vi "FL24 Dryer Tool Main.vi"() -> ()   [LabVIEW 2016]
uses:
  Common/LabVIEW GEA2 Toolkit/LabVIEW_GEA2_Toolkit.lvlibp/type defs/Data In.ctl
  Common/LabVIEW GEA2 Toolkit/LabVIEW_GEA2_Toolkit.lvlibp/type defs/Source_Destination.ctl
  Common/LabVIEW GEA2 Toolkit/LabVIEW_GEA2_Toolkit.lvlibp/type defs/Data Type.ctl
  Common/LabVIEW GEA2 Toolkit/LabVIEW_GEA2_Toolkit.lvlibp/type defs/ERD Read Data In.ctl
  Laundry Tool 2.0 Support/type defs2/Select _Graph_Brass.ctl
  Laundry Tool 1.0 Support/type defs/ERD_Graph_All.ctl
  Laundry Tool 1.0 Support/type defs/ERD_Graph.ctl
  Laundry Tool 1.0 Support/type defs/Version.ctl
  Laundry Tool 2.0 Support/type defs2/ERD_Always_Show_Brass.ctl
  Laundry Tool 1.0 Support/type defs/Fault_Buffer_Status.ctl
  Laundry Tool 2.0 Support/type defs2/Diagnostics_Table.ctl
  Laundry Tool 1.0 Support/type defs/Cycle_Diag_Buffer_Status.ctl
  Laundry Tool 2.0 Support/type defs2/ERD_Data_Loop_Control_Brass.ctl
  Laundry Tool 2.0 Support/type defs2/ERD_Loop_States_Brass.ctl
  Laundry Tool 2.0 Support/type defs2/Error_Command_Brass.ctl
  Laundry Tool 2.0 Support/type defs2/DAQ_States_Brass.ctl
  Common/GExplorer Support/typedefs/GExplorer_Data_Cluster.ctl
  Laundry Tool 1.0 Support/type defs/Cont_Send_States.ctl
  Laundry Tool 2.0 Support/type defs2/Cont_Send_States_Brass.ctl
  Common/LabVIEW GEA2 Toolkit/LabVIEW_GEA2_Toolkit.lvlibp/type defs/Data Out.ctl
  Common/LabVIEW GEA2 Toolkit/LabVIEW_GEA2_Toolkit.lvlibp/type defs/ERD Write Data In.ctl
  Laundry Tool 2.0 Support/type defs2/DAQ_Control_Command_Brass.ctl
  Laundry Tool 2.0 Support/type defs2/ERD_Loop_Control_Command_Brass.ctl
  Laundry Tool 2.0 Support/type defs2/GEA2_Control_Command_Brass.ctl
  <vilib>/DAQmx/read.llb/DAQmx Read (Digital 1D Bool NChan 1Samp 1Line).vi
  <vilib>/DAQmx/read.llb/DAQmx Read (Digital 1D U8 1Chan NSamp).vi
  <vilib>/DAQmx/write.llb/DAQmx Write (Digital Bool 1Line 1Point).vi
  <vilib>/DAQmx/read.llb/DAQmx Read (Counter U32 1Chan 1Samp).vi
  <vilib>/DAQmx/write.llb/DAQmx Write (Analog 1D DBL NChan 1Samp).vi
  <vilib>/DAQmx/write.llb/DAQmx Write (Digital 1D Bool NChan 1Samp 1Line).vi
  Common/LabVIEW GEA2 Toolkit/LabVIEW_GEA2_Toolkit.lvlibp/advanced/GEA2 Message Received Event Handler.vi
  <vilib>/DAQmx/create/channels.llb/DAQmx Create Channel (DO-Digital Output).vi
  <vilib>/DAQmx/create/channels.llb/DAQmx Create Channel (DI-Digital Input).vi
  <vilib>/DAQmx/configure/timing.llb/DAQmx Timing (Sample Clock).vi
  <vilib>/DAQmx/create/channels.llb/DAQmx Create Channel (CO-Pulse Generation-Frequency).vi
  <vilib>/DAQmx/configure/timing.llb/DAQmx Timing (Implicit).vi
  <vilib>/DAQmx/create/channels.llb/DAQmx Create Channel (CI-Count Edges).vi
  <vilib>/DAQmx/create/channels.llb/DAQmx Create Channel (AO-Voltage-Basic).vi
  <vilib>/DAQmx/miscellaneous.llb/DAQmx Fill In Error Info.vi
  C:/Automation/DLLs/PC Dot Net/GeaCommunication.dll
  Common/LabVIEW GEA2 Toolkit/LabVIEW_GEA2_Toolkit.lvlibp
  Automation/Product Specific/Clothes Care/2015 VA Washer/Projects/2015 VA Washer.lvlib
  <resource>/objmgr/daqmx.rc
panel:
  in  "Data ON":bool=TRUE
  out "ERD_Always Show":T1
  in  "Stop":bool
  out "Fault Status":bool
  out "Log Rate (ms)":u32
  in  "Tab Control":T2(tab)
  in  "Filter Data":bool=TRUE
  in  "Start Send":bool
  in  "Cmd":string
  in  "Filter Log":bool
  in  "Msg Rate (ms)":u32=1000 min=50 step=50
  out "CSV File Log Path":path=path "C:/Users/502129737/Desktop/1"
  in  "Clear":bool
  out "GEA2 Log":string
  in  "Board Index":u8 max=0 step=1
  out "Board ID":string="0"
  in  "GEA2 Send":T3={"Source"=228, "Destination"=53, "Command"=0, "Message"=""} {"Command" format="%02x"; "Destination" format="%02x"; "Source" format="%02x"}
  in  "Send Button":bool
  in  "GEA2 Log Length":i32=100000
  in  "Save Log":bool
  out "Version":T4
  in  "GEA Inputs":T5={"Source"=228, "Destination"=53} {"Destination" format="%.0x"; "Source" format="%.0x"}
  in  "Read ERD List":T6[](array[typedef])=[{"ERD Number"=0, "Data Type"=enum."string"}] {"ERD Number" format="%.0x"}
  out "Read ERD Data Out":cluster{"ERD Number":u16, "Data":string}[](array[cluster]) {"ERD Number" format="%.0x"}
  in  "Read ERD":bool
  in  "Write ERD":bool
  in  "Write ERD List":T8(array[cluster])=[{"ERD Number"=0, "Data Type"=enum."string", "Data"=""}] {"ERD Number" format="%.0x"}
  in  "Graphing ON":bool=TRUE
  in  "Select Graph":T9
  out "ERD 3":dbl(graph)
  out "ERD 2":dbl(graph)
  out "ERD 1":dbl(graph)
  out "All Loads":u16[][](graph)
  in  "ERD Graphing ON":bool
  out "ERD Graph  Ind":T10
  in  "ERD Graph Cntrl":T11={"ERD 3"={"ERD #"=142, "Data Type"=enum."uint32_t", "Scaler"=32}, "ERD 2"={"ERD #"=142, "Data Type"=enum."uint32_t", "Scaler"=32}, "ERD 1"={"ERD #"=142, "Data Type"=enum."int32_t", "Scaler"=32}} {"ERD 1"."Scaler" min=1; "ERD 1"."ERD #" format="%.0x"; "ERD 2"."Scaler" min=1; "ERD 2"."ERD #" format="%.0x"; "ERD 3"."Scaler" min=1; "ERD 3"."ERD #" format="%.0x"}
  in  "Save Fault Log":bool
  in  "Clear Fault Table Buffer":bool
  in  "Clear Fault Seq Buffer":bool
  in  "Fault ON":bool
  out "Fault Table Buffer":string[][](table)
  out "Fault Sequence Buffer":string
  out "Seq Buffer Status":T13
  out "Table Buffer Status":T13
  in  "Save Cycle History Log":bool
  in  "Clear Cycle Buffer":bool
  out "Cycle Buffer Status":T14
  in  "Get Cycle History":bool
  out "Diagnostics Table":T15
  in  "Test Mode":cluster{"Exit":bool, "Enter":bool}
  in  "Drum Light":cluster{"ON":bool, "OFF":bool}
  in  "Motor":cluster{"CW":bool, "OFF":bool, "CCW":bool}
  in  "Heaters":T16
  in  "Pump":cluster{"ON":bool, "OFF":bool}
  in  "Main Relay":cluster{"ON":bool, "OFF":bool}
  in  "Buzzer":cluster{"ON":bool, "OFF":bool}
  in  "LEDs":cluster{"ON":bool, "OFF":bool}
  in  "HE/LE ?":enum16{"HE", "LE"}(ring)
  in  "LL (M - A)":bool=TRUE
  in  "Lid Lock Feedback":bool
  in  "MS (M - A)":bool=TRUE
  out "DAQ Status":string
  out "Drain Pump":bool
  out "Mode Shift":bool
  out "Recirc Pump":bool
  out "Cold Valve":bool
  out "Hot Valve":bool
  out "Spray/Rinse Valve":bool
  out "Fabric SoftValve":bool
  in  "AC Power":bool=TRUE
  in  "Mode Shift FB":bool
  in  "Lid Status":bool=TRUE
  in  "Pressure":dbl(slide) min=0.0 max=5.0 step=0.5 scale=0.0..5.0 scale format="%#_3g"
  in  "Motor Current":dbl(slide)=2.5 min=0.0 max=5.0 step=0.5 scale=0.0..5.0 scale format="%#_3g"
  in  "Turn On DAQ":bool
  out "DAQ On?":bool
  in  "Basket RPM":dbl=1.0 min=1.0 max=800.0 step=5.0
  in  "Temperature":dbl(slide)=2.5 min=0.0 max=5.0 step=0.5 scale=0.0..5.0 scale format="%#_3g"
  out "Triac CW":bool
  out "Traic CCW":bool
  out "CCW":u32
  out "CW":u32
  in  "ERD Read List":T17(array[cluster])=[{"Boolean"=TRUE, "ERD Number"=1, "ERD Name"="Model Number", "Data Type"=enum."string"}, {"Boolean"=TRUE, "ERD Number"=2, "ERD Name"="Serial Number", "Data Type"=enum."string"}, {"Boolean"=TRUE, "ERD Number"=8192, "ERD Name"="Machine Status", "Data Type"=enum."uint8_t"}, {"Boolean"=TRUE, "ERD Number"=8202, "ERD Name"="Cycle Name", "Data Type"=enum."string"}, {"Boolean"=TRUE, "ERD Number"=142, "ERD Name"="Cycle Count", "Data Type"=enum."uint32_t"}, {"Boolean"=TRUE, "ERD Number"=8193, "ERD Name"="Sub-Cycle", "Data Type"=enum."string"}, {"Boolean"=TRUE, "ERD Number"=141, "ERD Name"="System Runtime", "Data Type"=enum."uint32_t"}, {"Boolean"=TRUE, "ERD Number"=8208, "ERD Name"="Delay Time", "Data Type"=enum."uint16_t"}, {"Boolean"=FALSE, "ERD Number"=256, "ERD Name"="Version", "Data Type"=enum."string"}, {"Boolean"=TRUE, "ERD Number"=70, "ERD Name"="Cycle Time", "Data Type"=enum."uint16_t"}, {"Boolean"=TRUE, "ERD Number"=8206, "ERD Name"="Operating Mode", "Data Type"=enum."string"}, {"Boolean"=TRUE, "ERD Number"=8217, "ERD Name"="Temp Level", "Data Type"=enum."string"}, {"Boolean"=TRUE, "ERD Number"=8218, "ERD Name"="Dryness Level", "Data Type"=enum."string"}, {"Boolean"=TRUE, "ERD Number"=8219, "ERD Name"="Extended Tumble", "Data Type"=enum."string"}, {"Boolean"=TRUE, "ERD Number"=61447, "ERD Name"="Input Status", "Data Type"=enum."string"}, {"Boolean"=TRUE, "ERD Number"=61448, "ERD Name"="Dryer Type", "Data Type"=enum."string"}, {"Boolean"=TRUE, "ERD Number"=8220, "ERD Name"="Cycle Type", "Data Type"=enum."string"}, {"Boolean"=TRUE, "ERD Number"=61449, "ERD Name"="Software Version", "Data Type"=enum."string"}] {"ERD Number" format="%.0x"}
  out "Error Out":errorcluster
  in  "Error In":errorcluster
  # "UI: 0x35\nMC: 0x2C"
  # "Software Version"
  # "UI - Critical Version"
  # "UI - Non-Critical"
  # "MC -  Version"
  # "Diagnostic Data Version"
  # "Model Setting"
  # "Heater Type"
  # "Must input a valid ERD# and Data Type\nDO NOT Leave Blank \nIf no scaler use value of 01"
  # "Contact:\n\nDerek Hibdon\nderek.hibdon@ge.com"
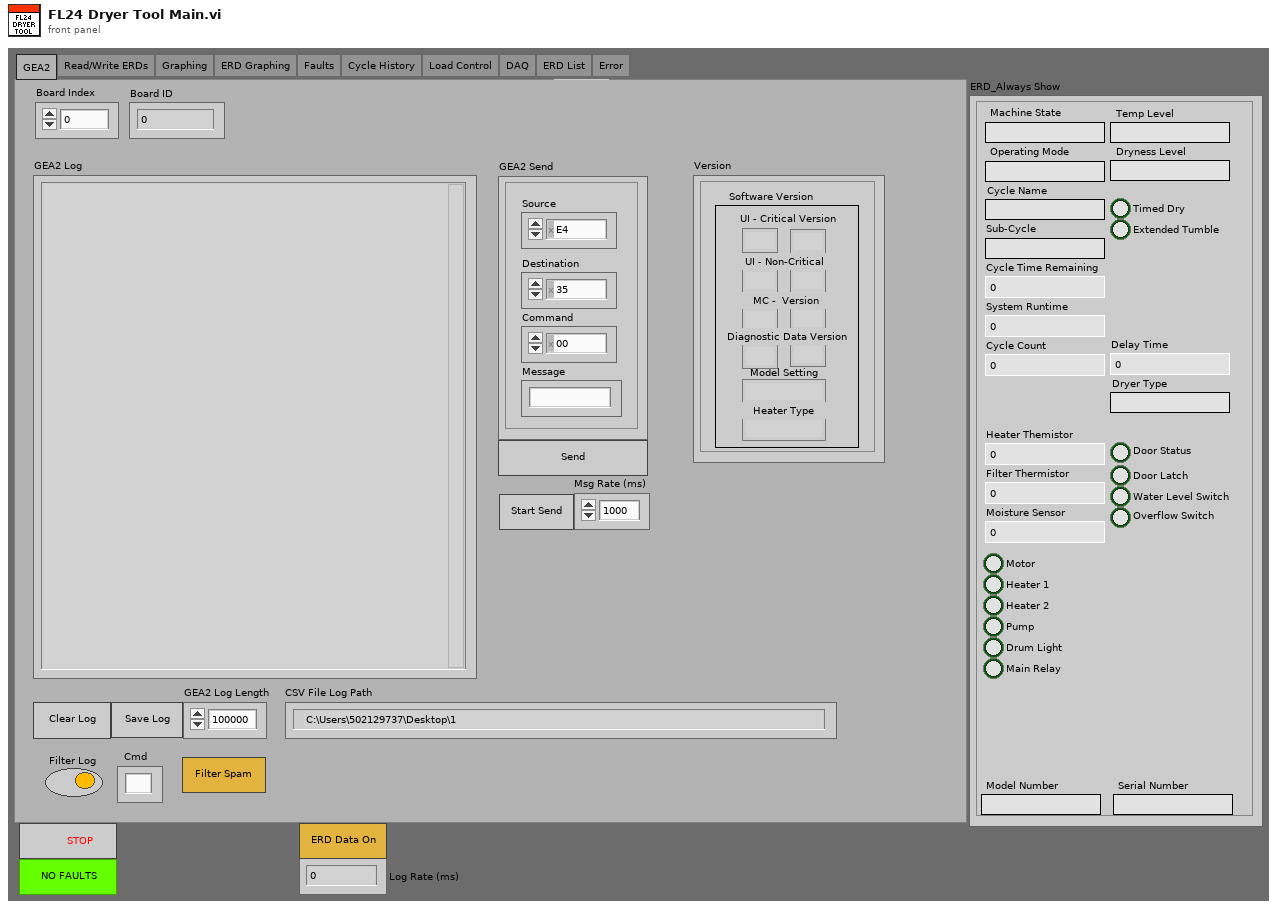
[diagram p1: front panel]
types:
  T1 = typedef "ERD_Always_Show_Brass.ctl" = cluster{"Machine State":string, "Cycle Count":u32, "Dryness Level":string, "Temp Level":string, "Delay Time":u16, "Sub-Cycle":string, "Cycle Name":string, "Model Number":string, "Serial Number":string, "System Runtime":u32, "Cycle Time Remaining":u16, "Operating Mode":string, "Heater Themistor":u16, "Water Level Switch":bool, "Overflow Switch":bool, "Door Status":bool, "Door Latch":bool, "Heater 1":bool, "Filter Thermistor":u16, "Moisture Sensor":u16, "Dryer Type":string, "Timed Dry":bool, "Extended Tumble":bool, "Heater 2":bool, "Pump":bool, "Drum Light":bool, "Main Relay":bool, "Motor":bool}
  T2 = enum32{"GEA2", "Read/Write ERDs", "Graphing", "ERD Graphing", "Faults", "Cycle History", "Load Control", "DAQ", "ERD List", "Error"}
  T3 = typedef "LabVIEW_GEA2_Toolkit.lvlibp/Data In.ctl" = cluster{"Source":u8, "Destination":u8, "Command":u8, "Message":string}
  T4 = typedef "Version.ctl" = cluster{"UI - Critical Major":string, "UI - Critical Minor":string, "UI - Non-Critical Minor":string, "UI - Non-Critical Major":string, "MC Minor":string, "MC Major":string, "Model Setting":string, "Diagnostic Data Minor":string, "Diagnostic Data Major":string, "Heater Type":string}
  T5 = typedef "LabVIEW_GEA2_Toolkit.lvlibp/Source_Destination.ctl" = cluster{"Source":u8, "Destination":u8}
  T6 = typedef "LabVIEW_GEA2_Toolkit.lvlibp/ERD Read Data In.ctl" = cluster{"ERD Number":u16, "Data Type":T7}
  T7 = typedef "LabVIEW_GEA2_Toolkit.lvlibp/Data Type.ctl" = enum16{"string", "boolean", "uint8_t", "uint16_t", "uint32_t", "uint64_t", "int8_t", "int16_t", "int32_t", "int64_t"}
  T8 = cluster{"ERD Number":u16, "Data Type":T7, "Data":string}[]
  T9 = typedef "Select _Graph_Brass.ctl" = enum16{"All Loads", "ERD 1", "ERD 2", "ERD 3", "Temperature (F)", "Basket Speed (RPM)", "Tub Volume (Gal)", "Pressure (in H2O)", "Current RMS (Amps)"}
  T10 = cluster{"ERD Value 1":dbl, "ERD Value 2":dbl, "ERD Value 3":dbl}
  T11 = typedef "ERD_Graph_All.ctl" = cluster{"ERD 3":T12, "ERD 2":T12, "ERD 1":T12}
  T12 = typedef "ERD_Graph.ctl" = cluster{"ERD #":u16, "Data Type":T7, "Scaler":u32}
  T13 = typedef "Fault_Buffer_Status.ctl" = cluster{"Current Index":u16, "Count":u16, "Overwrite Count":u16}
  T14 = typedef "Cycle_Diag_Buffer_Status.ctl" = cluster{"Current Index":u16, "Count":u16, "Overwrite Count":u16}
  T15 = typedef "Diagnostics_Table.ctl" = string[][]
  T16 = cluster{"Heater 1":bool, "BOTH":bool, "Heater 2":bool, "OFF":bool}
  T17 = cluster{"Boolean":bool, "ERD Number":u16, "ERD Name":string, "Data Type":enum16{"string", "boolean", "uint8_t", "uint16_t", "uint32_t", "uint64_t"}}[]
  T18 = typedef "Cont_Send_States_Brass.ctl" = enum16{"Run", "Shutdown"}
  T19 = typedef "Cont_Send_States.ctl" = enum16{"Run", "Shutdown"}
  T20 = typedef "GExplorer_Data_Cluster.ctl" = cluster{"Data":variant, "State":enum16{"Add to Log", "Clear", "Shutdown"}}
  T21 = typedef "DAQ_States_Brass.ctl" = enum16{"Wait for Init", "Rename Devices", "Verify Hardware", "Initialize", "Run", "Shutdown", "Exit"}
  T22 = typedef "ERD_Data_Loop_Control_Brass.ctl" = cluster{"Data":variant, "State":T23}
  T23 = typedef "ERD_Loop_States_Brass.ctl" = enum16{"Init", "Build ERD Read List", "Read ERDs", "Update UI", "Update Graphs", "Read Faults", "Log Data", "Pause", "Shutdown"}
  T24 = typedef "Error_Command_Brass.ctl" = enum16{"Initialize", "Handle Errors", "Report Errors"}
  T25 = typedef "LabVIEW_GEA2_Toolkit.lvlibp/ERD Write Data In.ctl" = cluster{"ERD Number":u16, "Data Type":T7, "Data":string}
  T26 = typedef "GEA2_Control_Command_Brass.ctl" = enum16{"Initialize", "Shutdown"}
  T27 = typedef "ERD_Loop_Control_Command_Brass.ctl" = enum16{"Initialize", "Shutdown"}
  T28 = typedef "DAQ_Control_Command_Brass.ctl" = enum16{"Initialize", "Shutdown", "Exit"}
  T29 = enum8{"Enabled", "Disabled", "Disabled and Grayed Out"}
  T30 = typedef "LabVIEW_GEA2_Toolkit.lvlibp/Data Out.ctl" = cluster{"Source":u8, "Destination":u8, "Command":u8, "Length":u8, "CRC":u16, "Message":string}
  T31 = typedef "LabVIEW_GEA2_Toolkit.lvlibp/ERD Read Data Out.ctl" = cluster{"ERD Number":u16, "Data":string}
  T32 = typedef "All_Bundled_Data_Brass.ctl" = cluster{"Version":T4, "ERD_Always Show":T1, "Personality Set":u8, "CSV File String Arrays":T33, "Fault Table Array ":T34}
  T33 = typedef "CSV_File_String_Arrays.ctl" = cluster{"ERD Number Array":string[], "ERD Name Array":string[], "ERD Converted String Data":string[]}
  T34 = typedef "Fault Table Array.ctl" = T35[]
  T35 = typedef "Fault_Table_Info.ctl" = cluster{"Cycle Count":u32, " Runtime (min) ":u32, "Fault Status":string, "Fault ID":string, "Fault Count":u16}
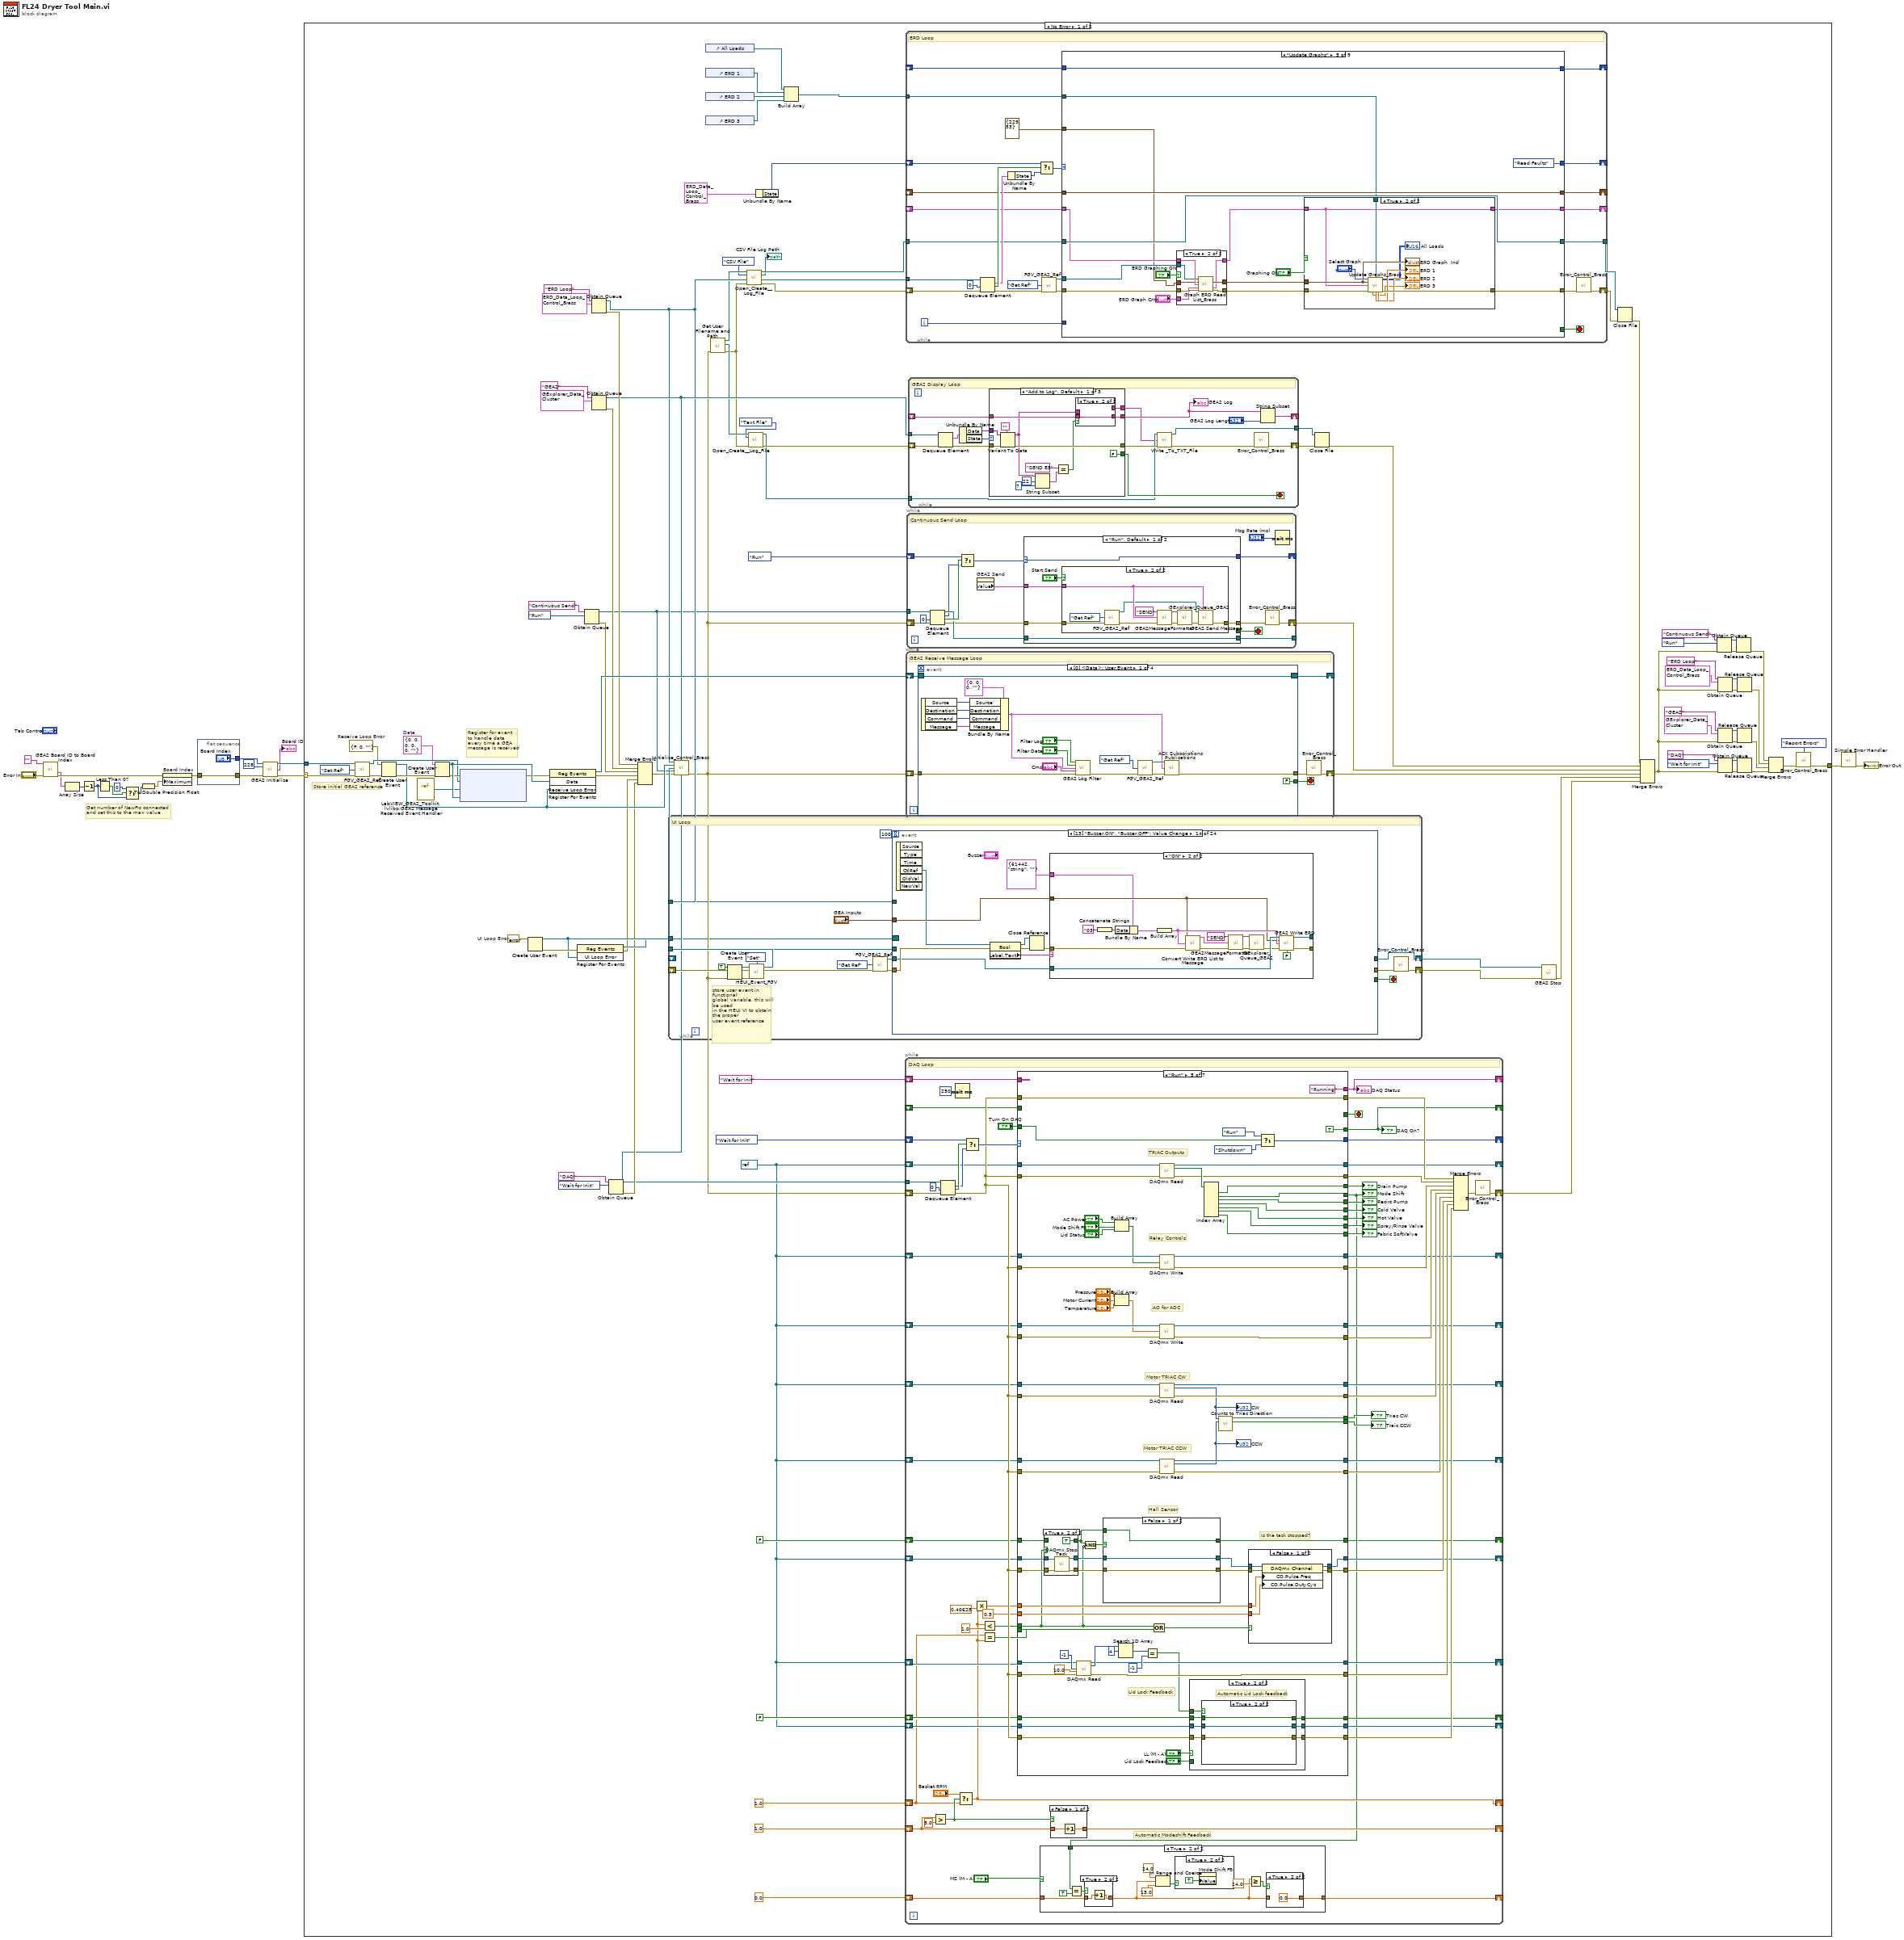
[diagram p0: block diagram]
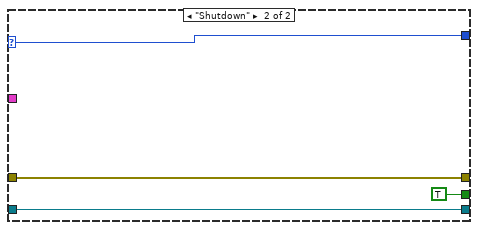
[diagram p3: hidden frame]
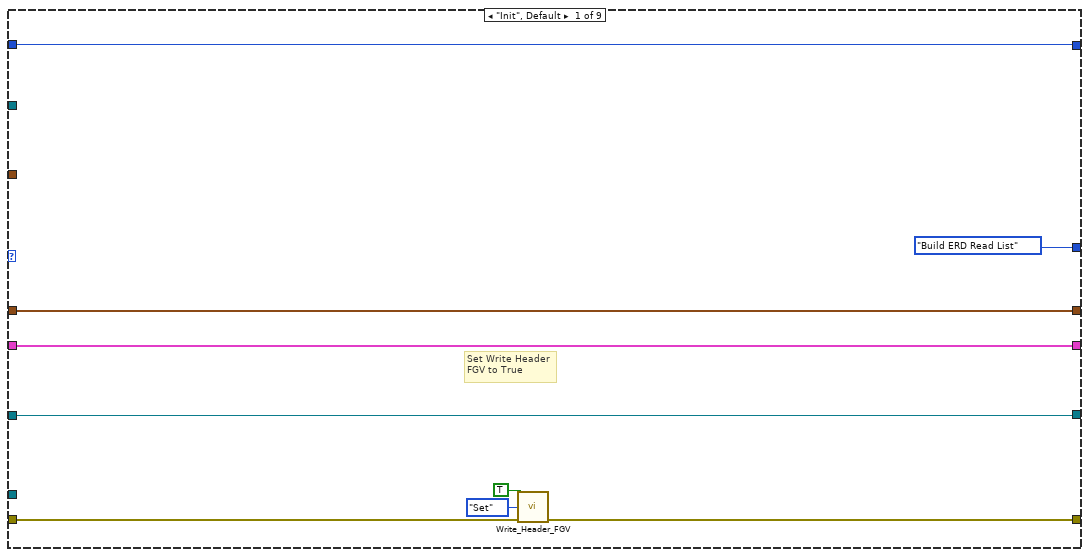
[diagram p4: hidden frame]
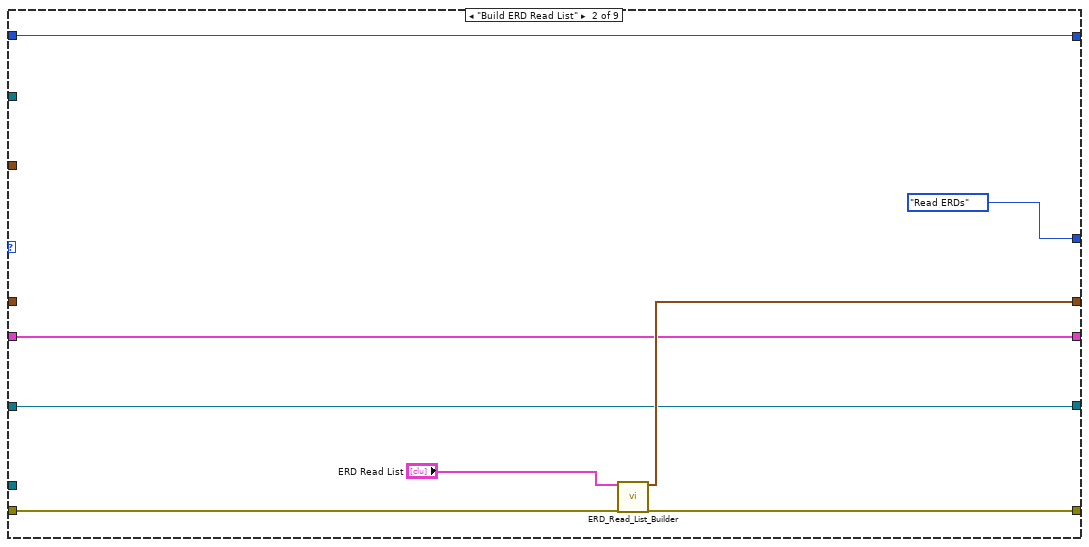
[diagram p5: hidden frame]
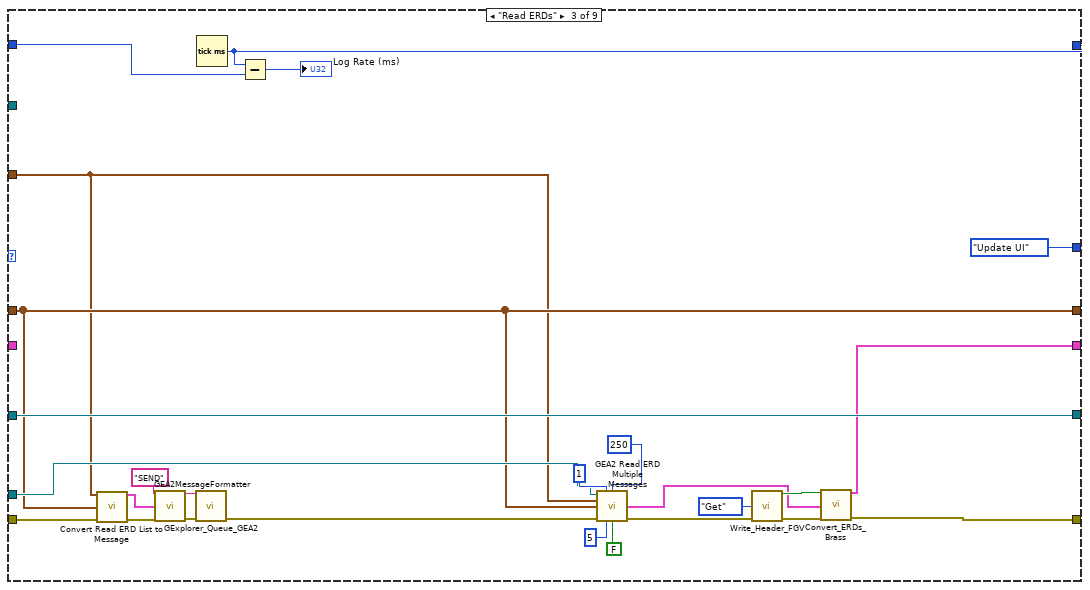
[diagram p6: hidden frame]
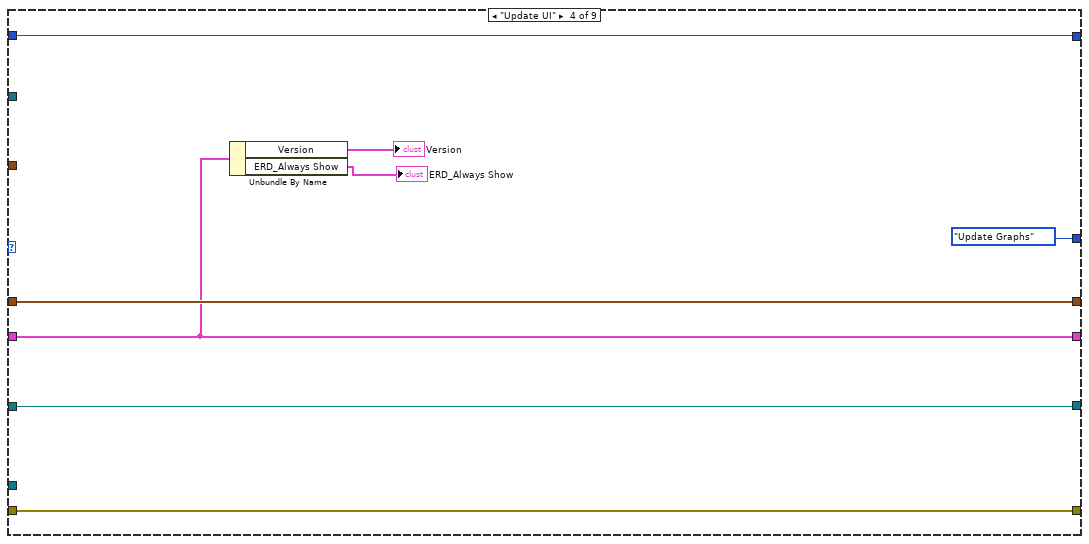
[diagram p7: hidden frame]
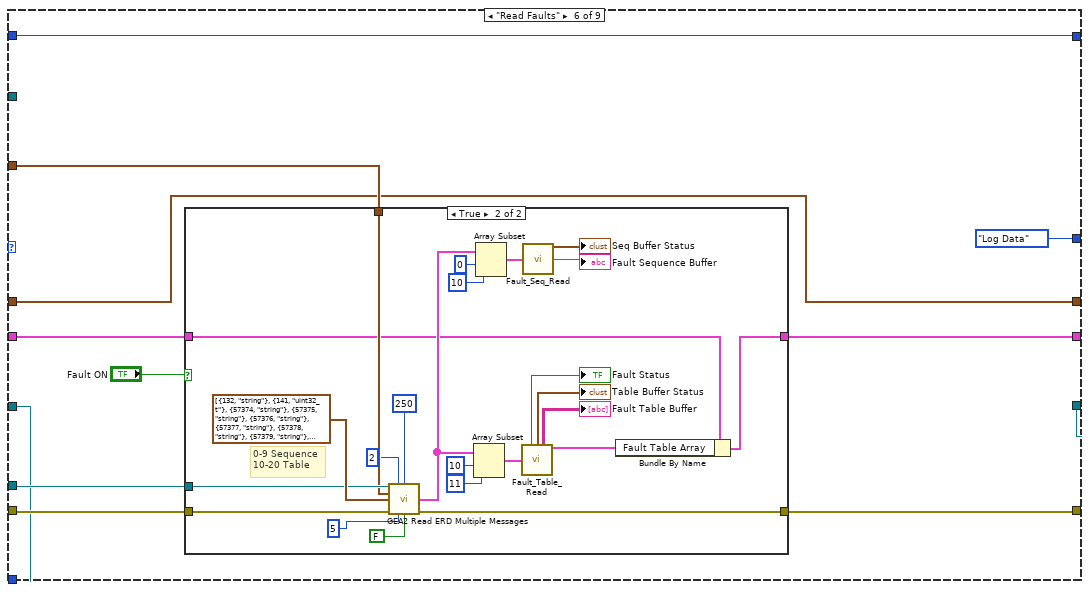
[diagram p10: hidden frame]
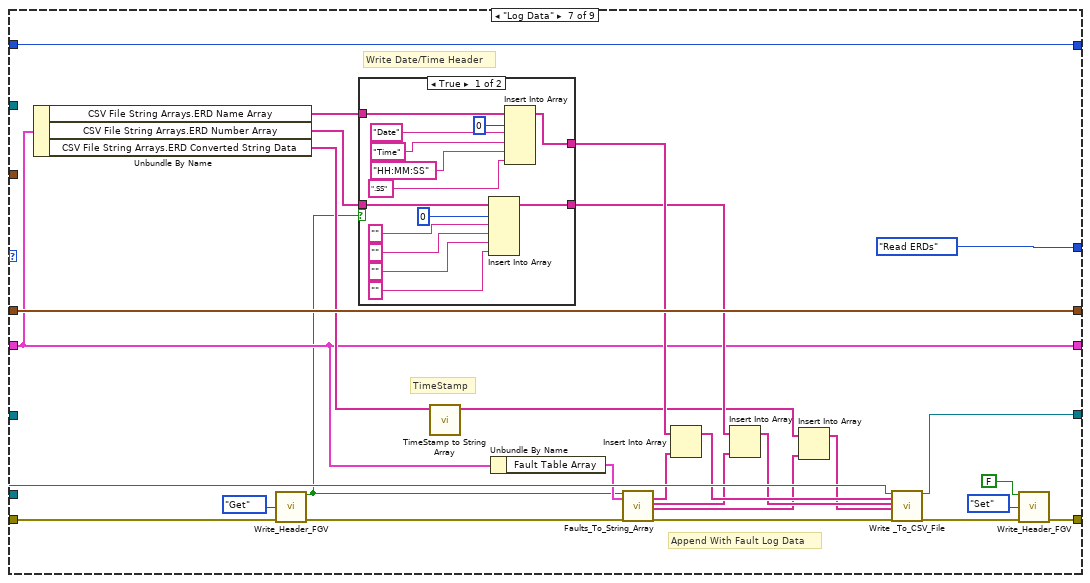
[diagram p12: hidden frame]
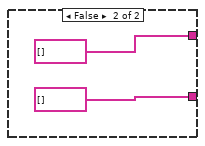
[diagram p13: hidden frame]
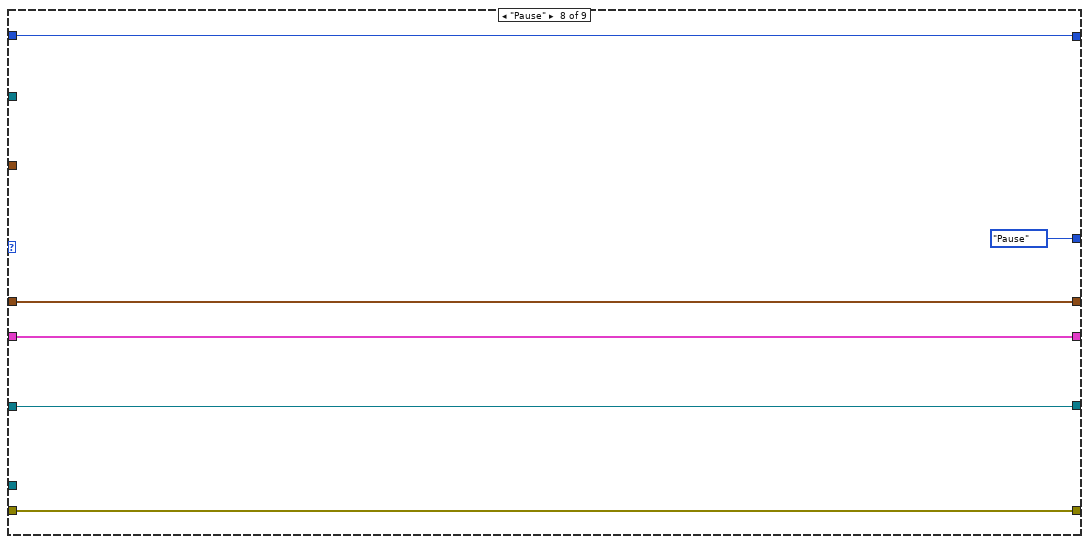
[diagram p14: hidden frame]
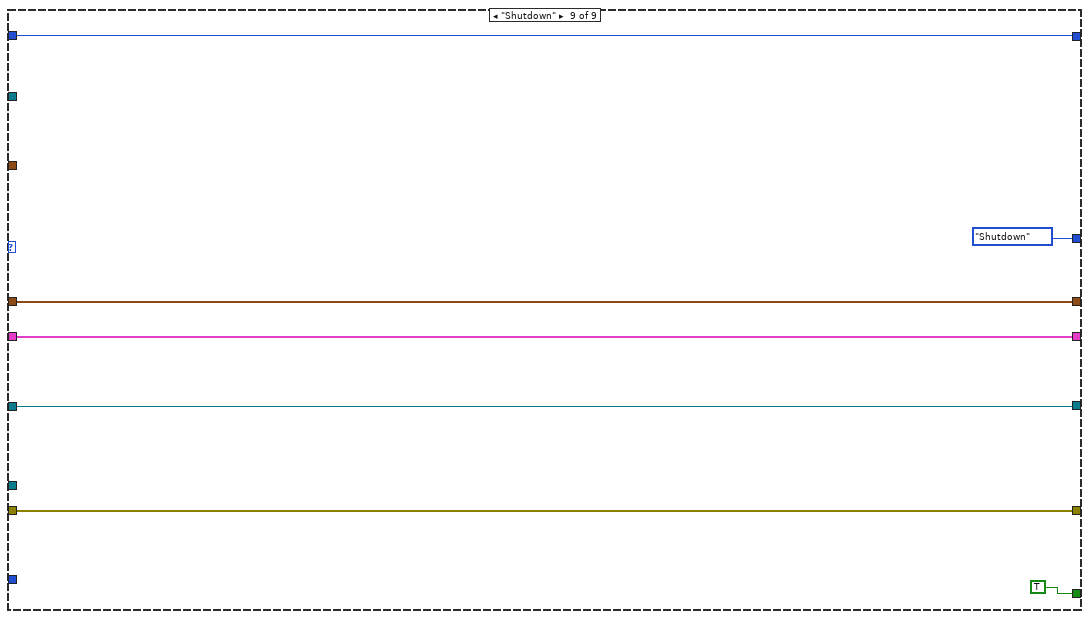
[diagram p15: hidden frame]
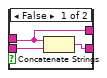
[diagram p16: hidden frame]
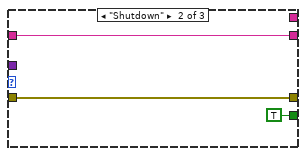
[diagram p17: hidden frame]
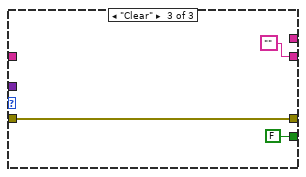
[diagram p18: hidden frame]
diagram:
  # "Get number of NewFIs connected\nand set this to the max value"
  n1 = call "GEA2 Board ID to Board Index.vi"("Board ID"="", "Error In"="Error In") -> ("Boards Found"=w4:string[], "Error Out"=w13:errorcluster)  [unwired: 9 in, 3 out]
  n2 = Array Size(array=w4) -> (size(s)=w9:i32)
  n3 = Decrement(x=w9) -> (x-1=w7:i32)
  n4 = Less Than 0?(x=w7) -> (x < 0?=w8:bool)
  n5 = Select(t=0, s=w8, f=w7) -> (s? t:f=w5:i32)
  n6 = To Double Precision Float(number=w5) -> (double precision float=w3:dbl)
  n7 = property on="Board Index" class="DigNum (strict)"(error in=w13, "Maximum"=w3) -> (error out=w11:errorcluster)  [unwired: 1 in, 1 out]
  n8 = flat-sequence {
    tunnel: ["Board Index"] -> w16
    tunnel: w11 -> [w20]
    tunnel: [w20] -> w10
    frame #0 {
    }
  }
  n9 = call "GEA2 Initialize.vi"("Board Index"=w16, "Source Address"=u8 228, "error in"=w10) -> ("GEA2 Reference Out"=w18:refnum<k24>, "Board ID"=→"Board ID":string, "error out"=w17:errorcluster)  [unwired: 10 in]
  n10 = case shown="No Error" w17 {
    selector: w17 -> [w81 w1659]
    tunnel: w18 -> [w79 _]
    tunnel: [w83 w1659] -> w2
    frame No Error {
      w35 = errorcluster {"status"=FALSE, "code"=0, "source"=""}  # Receive Loop Error
      w36 = T30 {"Source"=0, "Destination"=0, "Command"=0, "Length"=0, "CRC"=0, "Message"=""}  # Data
      w51 = refnum<k21> refnum ("task out")
      w117 = errorcluster {"status"=FALSE, "code"=0, "source"=""}  # UI Loop Error
      # "store user event in functional\nglobal variable, this will be used\nin the HEUI VI to obtain the proper\nuser event reference"
      # "Store initial GEA2 reference"
      # "Register for event\nto handle data\nevery time a GEA\nmessage is received"
      n11 = call "FGV_GEA2_Ref.vi"("GEA2 Reference In"=w79, "Action"=enum16{"Set Ref", "Get Ref"}."Set Ref", "Error In"=w81) -> ("GEA2 Reference Out"=w78:refnum<k24>, "Error Out"=w80:errorcluster)  [unwired: 11 in]
      n12 = Create User Event(user event datatype=w35, error in=w80) -> (user event=w118:refnum<user-event>, error out=w120:errorcluster)
      n13 = vi-ref "LabVIEW_GEA2_Toolkit.lvlibp:GEA2 Message Received Event Handler.vi"() -> (w119:refnum<vi>)
      n14 = Create User Event(user event datatype=w36, error in=w120) -> (user event=w123:refnum<user-event>, error out=w122:errorcluster)
      n15 = node(w122, w78, w119, w123) -> (w121:errorcluster)  [unwired: 1 in, 1 out]
      n16 = Create User Event(user event datatype=w117) -> (user event=w106:refnum<user-event>, error out=w116:errorcluster)  [unwired: 1 in]
      n17 = register-events(error in=w121, w123, w118) -> (reference out=w115:refnum<event-registration>, error out=w88:errorcluster)  [unwired: 1 in]
      n18 = register-events(error in=w116, w106) -> (reference out=w97:refnum<event-registration>, error out=w87:errorcluster)  [unwired: 1 in]
      n19 = Obtain Queue(name (unnamed)="Continuous Send", element data type=Cont_Send_States_Brass."Run" ("State")) -> (queue out=w37:refnum<queue>, error out=w42:errorcluster)  [unwired: 3 in, 1 out]
      n20 = Obtain Queue(name (unnamed)="ERD Loop", element data type=T22 {"Data"=variant, "State"=enum."Read ERDs"} ("Data")) -> (queue out=w66:refnum<queue>, error out=w84:errorcluster)  [unwired: 3 in, 1 out]
      n21 = Obtain Queue(name (unnamed)="GEA2", element data type=T20 {"Data"=variant, "State"=enum."Add to Log"} ("Data")) -> (queue out=w67:refnum<queue>, error out=w89:errorcluster)  [unwired: 3 in, 1 out]
      n22 = Obtain Queue(name (unnamed)="DAQ", element data type=DAQ_States_Brass."Wait for Init" ("States")) -> (queue out=w59:refnum<queue>, error out=w86:errorcluster)  [unwired: 3 in, 1 out]
      n23 = Merge Errors(w84, w89, w42, w88, w87, w86) -> (w85:errorcluster)
      n24 = call "Initialize_Control_Brass.vi"("ERD Loop"=w66, "GEA2"=w67, "Receive Loop"=w118, "UI Loop Error"=w106, "Cont Send"=w37, "Error In"=w85, "DAQ"=w59) -> ("Error Out"=w32:errorcluster)  [unwired: 8 in]
      n25 = control-ref of="All Loads"() -> (w22:refnum<vi>)
      n26 = control-ref of="ERD 1"() -> (w63:refnum<vi>)
      n27 = control-ref of="ERD 2"() -> (w61:refnum<vi>)
      n28 = control-ref of="ERD 3"() -> (w62:refnum<vi>)
      n29 = call "Get User Filename and Path.vi"("error in (no error)"=w32) -> ("error out"=w24:errorcluster, "TXT File Path"=w30:path, "CSV File Path"=w33:path)  [unwired: 8 in]
      n30 = Create User Event(user event datatype=TRUE ("Bool"), error in=w32) -> (user event=w73:refnum<user-event>, error out=w74:errorcluster)
      n31 = call "Open_Create__Log_File.vi"("File Path Control"=w33, "Enum"=enum16{"CSV File", "Text File"}."CSV File", "Error In"=w24) -> ("refnum out"=w64:refnum<file>, "File Path"=→"CSV File Log Path":path, "Error Out"=w76:errorcluster)  [unwired: 10 in]
      n32 = call "Open_Create__Log_File.vi"("File Path Control"=w30, "Enum"=enum16{"CSV File", "Text File"}."Text File", "Error In"=w24) -> ("refnum out"=w29:refnum<file>, "Error Out"=w31:errorcluster)  [unwired: 10 in, 1 out]
      n33 = call "HEUI_Event_FGV.vi"("Event In"=w73, "Action"=enum16{"Get", "Set"}."Set", "Error In"=w74) -> ("Event Out"=w70:refnum<user-event>, "Error Out"=w71:errorcluster)  [unwired: 11 in]
      n34 = while "UI Loop" {
        shift-right: [w1014] -> w125
        shift-left: w71 -> [w1008]
        shift-right: [w1016] -> w124
        shift-left: _ -> [_]
        tunnel: w97 -> [w1015]
        tunnel: w70 -> [w1005]
        tunnel: w66 -> [w1004]
        stop <- w1013 stop-if-true
        # "UI Loop"
        n35 = call "FGV_GEA2_Ref.vi"("Action"=enum16{"Set Ref", "Get Ref"}."Get Ref", "Error In"=w1008) -> ("GEA2 Reference Out"=w1007:refnum<k24>, "Error Out"=w1009:errorcluster)  [unwired: 12 in]
        n36 = event shown="[13] \"Buzzer.ON\", \"Buzzer.OFF\": Value Change" {
          selector: w1015 -> [_ _ _ _ _ _ _ _ _ _ _ _ _ _ _ _ _ _ _ _ _ _ _ _]
          dyn-events: _ -> [_ _ _ _ _ _ _ _ _ _ _ _ _ _ _ _ _ _ _ _ _ _ _ _]
          timeout: 100 -> [_ _ _ _ _ _ _ _ _ _ _ _ _ _ _ _ _ _ _ _ _ _ _ _]
          tunnel: [w1022 w1032 w1033 w1039 w1053 w1063 w1076 w1083 w1086 w1105 _ _ _ _ _ _ _ _ w1517 w1536 w1550 w1568 w1588 w1599] -> w1012
          tunnel: w1009 -> [w1019 w1029 w1033 w1035 w1050 w1067 w1074 w1081 w1090 w1108 w1123 w1166 w1209 w1252 w1295 w1338 w1398 w1475 w1520 w1542 w1558 w1574 w1589 w1606]
          tunnel: [_ _ _ _ _ _ _ _ _ _ _ _ _ _ _ _ _ _ _ _ _ _ _ TRUE] -> w1013
          tunnel: w1007 -> [w1017 w1031 w1034 w1037 w1051 _ _ _ w1092 w1107 w1122 w1165 w1208 w1251 w1294 w1337 w1397 w1474 w1519 w1541 w1552 w1573 _ w1609]
          tunnel: [w1024 w1031 w1034 w1040 w1052 _ _ _ _ w1106 _ _ _ _ _ _ _ _ w1518 _ _ _ _ w1609] -> w1016
          tunnel: "GEA Inputs" -> [_ _ _ w1038 w1048 _ _ _ w1091 w1109 w1121 w1164 w1207 w1250 w1293 w1336 w1396 w1473 w1521 w1539 w1551 w1575 _ _]
          tunnel: w1005 -> [_ _ _ _ _ _ _ _ _ _ _ _ _ _ _ _ _ _ _ _ _ _ _ _]
          tunnel: w1004 -> [_ _ _ _ _ _ w1072 w1079 _ _ _ _ _ _ _ _ _ _ _ _ _ _ w1586 _]
          event "Send Button": Value Change {
            n37 = event-data() -> ()  [unwired: 1 in, 1 out]
            n38 = call "GEA2MessageFormatter.vi"("Prefix(Send/Recv)"="SEND", "GEA2 Data In"="GEA2 Send", "Error In"=w1019) -> ("Output String"=w1021:string, "Error Out"=w1020:errorcluster)  [unwired: 11 in]
            n39 = call "GExplorer_Queue_GEA2.vi"("Output String"=w1021, "error in (no error)"=w1020) -> ("error out"=w1023:errorcluster)  [unwired: 13 in]
            n40 = call "GEA2 Send Message.vi"("GEA2 Reference In"=w1017, "Input Data"="GEA2 Send", "Error In"=w1023) -> ("GEA2 Reference Out"=w1024:refnum<k24>, "Error Out"=w1022:errorcluster)  [unwired: 11 in]
          }
          event "Clear": Value Change {
            w1026 = T20 {"Data"=variant, "State"=enum."Clear"} ("element")
            n41 = event-data() -> ()  [unwired: 1 in, 6 out]
            n42 = Obtain Queue(name (unnamed)="GEA2", element data type=w1026, error in (no error)=w1029) -> (queue out=w1027:refnum<queue>, error out=w1030:errorcluster)  [unwired: 2 in, 1 out]
            n43 = Enqueue Element(queue=w1027, element=w1026, error in (no error)=w1030) -> (error out=w1032:errorcluster)  [unwired: 1 in, 2 out]
          }
          event Timeout {
            # "Must have timeout case to give GEA2 FGV a chance to update\nthe GEA2 reference. Otherwise, when we receive an event it may\nbe using a reference that is no longer valid."
            n44 = event-data() -> ()  [unwired: 1 in, 3 out]
          }
          event "Write ERD": Value Change {
            n45 = event-data() -> ()  [unwired: 1 in, 1 out]
            n46 = call "Convert Write ERD List to Message.vi"("GEA Inputs"=w1038, "Write ERD List"="Write ERD List", "Error In"=w1035) -> ("GEA Message"=w1044:T3, "Error Out"=w1045:errorcluster)  [unwired: 11 in]
            n47 = call "GEA2MessageFormatter.vi"("Prefix(Send/Recv)"="SEND", "GEA2 Data In"=w1044, "Error In"=w1045) -> ("Output String"=w1046:string, "Error Out"=w1047:errorcluster)  [unwired: 11 in]
            n48 = call "GExplorer_Queue_GEA2.vi"("Output String"=w1046, "error in (no error)"=w1047) -> ("error out"=w1042:errorcluster)  [unwired: 13 in]
            n49 = call "GEA2 Write ERD.vi"("GEA2 Reference In"=w1037, "GEA Inputs"=w1038, "Write ERD List"="Write ERD List", "Error In"=w1042, "Verify ERD Response?"=FALSE) -> ("GEA2 Reference Out"=w1040:refnum<k24>, "Error Out"=w1039:errorcluster)  [unwired: 8 in, 1 out]
          }
          event "Read ERD": Value Change {
            n50 = event-data() -> ()  [unwired: 1 in, 6 out]
            n51 = call "Convert Read ERD List to Message.vi"("GEA Inputs"=w1048, "Read ERD List"="Read ERD List", "Error In"=w1050) -> ("GEA Message"=w1058:T3, "Error Out"=w1049:errorcluster)  [unwired: 11 in]
            n52 = call "GEA2MessageFormatter.vi"("Prefix(Send/Recv)"="SEND", "GEA2 Data In"=w1058, "Error In"=w1049) -> ("Output String"=w1056:string, "Error Out"=w1055:errorcluster)  [unwired: 11 in]
            n53 = call "GExplorer_Queue_GEA2.vi"("Output String"=w1056, "error in (no error)"=w1055) -> ("error out"=w1059:errorcluster)  [unwired: 13 in]
            n54 = call "GEA2 Read ERD.vi"("GEA2 Reference In"=w1051, "GEA Inputs"=w1048, "Read ERD List"="Read ERD List", "Error In"=w1059, "Verify ERD Response?"=FALSE) -> ("GEA2 Reference Out"=w1052:refnum<k24>, "ERD Data Out"=→"Read ERD Data Out":T31[], "Error Out"=w1053:errorcluster)  [unwired: 7 in, 1 out]
          }
          event "Save Log": Value Change {
            n55 = event-data() -> ()  [unwired: 1 in, 6 out]
            n56 = property on="GEA2 Log" class="Str"(error in=w1067) -> (error out=w1069:errorcluster, "Value"=w1068:string)  [unwired: 1 in, 1 out]
            n57 = Write to Text File(prompt (Choose or enter file path)="Choose filename and path to save txt file to ", text=w1068, error in=w1069) -> (refnum out=w1066:refnum<file>, error out=w1065:errorcluster)  [unwired: 1 in, 1 out]
            n58 = Close File(refnum=w1066, error in=w1065) -> (error out=w1064:errorcluster)  [unwired: 1 out]
            n59 = call <vilib>:"Clear Errors.vi"("error in (no error)"=w1064, "specific error code to clear (0: all)"=43) -> ("error out"=w1063:errorcluster)  [unwired: 4 in, 1 out]
          }
          event "ERD Read List": Value Change {
            n60 = event-data() -> ()  [unwired: 1 in, 6 out]
            n61 = Enqueue Element(queue=w1072, element=T22 {"Data"=variant, "State"=enum."Build ERD Read List"}, error in (no error)=w1074) -> (error out=w1073:errorcluster)  [unwired: 1 in, 2 out]
            n62 = call "Write_Header_FGV.vi"("Write Header ? In"=TRUE, "Action"=enum16{"Get", "Set"}."Set", "Error In"=w1073) -> ("Error Out"=w1076:errorcluster)  [unwired: 11 in, 1 out]
          }
          event "Fault ON", "ERD Graphing ON": Value Change {
            n63 = event-data() -> ()  [unwired: 1 in, 6 out]
            n64 = Enqueue Element(queue=w1079, element=T22 {"Data"=variant, "State"=enum."Build ERD Read List"}, error in (no error)=w1081) -> (error out=w1080:errorcluster)  [unwired: 1 in, 2 out]
            n65 = call "Write_Header_FGV.vi"("Write Header ? In"=TRUE, "Action"=enum16{"Get", "Set"}."Set", "Error In"=w1080) -> ("Error Out"=w1083:errorcluster)  [unwired: 11 in, 1 out]
          }
          event "Save Fault Log": Value Change {
            # "0-16 Sequence\n17-27 Table"
            n66 = event-data() -> ()  [unwired: 1 in, 6 out]
            n67 = call "GEA2 Read ERD Multiple Messages.vi"("GEA2 Reference In"=w1092, "Read Timeout (ms)"=u32 250, "GEA Inputs"=w1091, "Read ERD List"=T6[] [{"ERD Number"=132, "Data Type"=enum."string"}, {"ERD Number"=141, "Data Type"=enum."uint32_t"}, {"ERD Number"=57394, "Data Type"=enum."string"}, {"ERD Number"=57395, "Data Type"=enum."string"}, {"ERD Number"=57396, "Data Type"=enum."string"}, {"ERD Number"=57397, "Data Type"=enum."string"}, {"ERD Number"=57398, "Data Type"=enum."string"}, {"ERD Number"=57399, "Data Type"=enum."string"}, {"ERD Number"=57400, "Data Type"=enum."string"}, {"ERD Number"=57401, "Data Type"=enum."string"}, {"ERD Number"=57402, "Data Type"=enum."string"}, {"ERD Number"=57403, "Data Type"=enum."string"}, {"ERD Number"=57404, "Data Type"=enum."string"}, {"ERD Number"=57405, "Data Type"=enum."string"}, {"ERD Number"=57406, "Data Type"=enum."string"}, {"ERD Number"=57407, "Data Type"=enum."string"}, {"ERD Number"=57408, "Data Type"=enum."string"}, {"ERD Number"=129, "Data Type"=enum."string"}, {"ERD Number"=57444, "Data Type"=enum."string"}, {"ERD Number"=57445, "Data Type"=enum."string"}, {"ERD Number"=57446, "Data Type"=enum."string"}, {"ERD Number"=57447, "Data Type"=enum."string"}, {"ERD Number"=57448, "Data Type"=enum."string"}, {"ERD Number"=57449, "Data Type"=enum."string"}, {"ERD Number"=57450, "Data Type"=enum."string"}, {"ERD Number"=57451, "Data Type"=enum."string"}, {"ERD Number"=57452, "Data Type"=enum."string"}, {"ERD Number"=57453, "Data Type"=enum."string"}], "Error In"=w1090, "#ERDs per message"=14 ("#ERDs per message 2"), "Verify ERD Response?"=FALSE) -> ("ERD Data Out"=w1095:T31[], "Error Out"=w1087:errorcluster)  [unwired: 5 in, 2 out]
            n68 = Array Subset(array=w1095, index=17, length=10) -> (w1096:T31[])
            n69 = Array Subset(array=w1095, index=0, length=17) -> (w1094:T31[])
            n70 = call "Fault_Seq_Read.vi"("Seq ERD In"=w1094) -> ("String"=w1089:string)  [unwired: 13 in, 1 out]
            n71 = call "Fault_Table_Read.vi"("ERD Data Out"=w1096) -> ("Fault Table String Out"=w1088:string[][])  [unwired: 11 in, 3 out]
            n72 = call "Fault_Logging.vi"("String"=w1089, "Fault Table String Out"=w1088, "error in (no error)"=w1087) -> ("error out"=w1086:errorcluster)  [unwired: 12 in]
          }
          event "Clear Fault Seq Buffer": Value Change {
            n73 = event-data() -> ()  [unwired: 1 in, 6 out]
            n74 = Bundle By Name(cluster=T25 {"ERD Number"=133, "Data Type"=enum."string", "Data"=""} ("ERD Read Data In"), "Data"="FF") -> (w1118:T25)
            n75 = Build Array(w1118) -> (w1112:T25[])
            n76 = call "Convert Write ERD List to Message.vi"("GEA Inputs"=w1109, "Write ERD List"=w1112, "Error In"=w1108) -> ("GEA Message"=w1114:T3, "Error Out"=w1115:errorcluster)  [unwired: 11 in]
            n77 = call "GEA2MessageFormatter.vi"("Prefix(Send/Recv)"="SEND", "GEA2 Data In"=w1114, "Error In"=w1115) -> ("Output String"=w1116:string, "Error Out"=w1117:errorcluster)  [unwired: 11 in]
            n78 = call "GExplorer_Queue_GEA2.vi"("Output String"=w1116, "error in (no error)"=w1117) -> ("error out"=w1113:errorcluster)  [unwired: 13 in]
            n79 = call "GEA2 Write ERD.vi"("GEA2 Reference In"=w1107, "Read Timeout (ms)"=u32 2000, "GEA Inputs"=w1109, "Write ERD List"=w1112, "Error In"=w1113, "Verify ERD Response?"=FALSE) -> ("GEA2 Reference Out"=w1106:refnum<k24>, "Error Out"=w1105:errorcluster)  [unwired: 7 in, 1 out]
          }
          event "Drum Light.ON", "Drum Light.OFF": Value Change {
            n80 = event-data() -> ("CtlRef"=w1120:refnum<vi>)  [unwired: 1 in, 5 out]
            n81 = property class="Bool"(reference=w1120, error in=w1123) -> (reference out=w1126:refnum<vi>, error out=w1127:errorcluster, "Label.Text"=w1128:string)
            n82 = Close Reference(reference=w1126, error in (no error)=w1127) -> (error out=w1125:errorcluster)
            n83 = case shown="\"ON\"" w1128 {
              tunnel: [w1133 w1159] -> _
              tunnel: w1122 -> [w1134 w1158]
              tunnel: w1125 -> [w1135 w1150]
              tunnel: w1121 -> [w1132 w1149]
              tunnel: [w1131 w1148] -> _
              tunnel: T25 {"ERD Number"=61441, "Data Type"=enum."string", "Data"=""} ("ERD Read Data In") -> [w1129 w1146]
              frame "OFF", Default {
                n84 = Concatenate Strings("00" ("string")) -> (w1145:string)
                n85 = Bundle By Name(cluster=w1129, "Data"=w1145) -> (w1144:T25)
                n86 = Build Array(w1144) -> (w1137:T25[])
                n87 = call "Convert Write ERD List to Message.vi"("GEA Inputs"=w1132, "Write ERD List"=w1137, "Error In"=w1135) -> ("GEA Message"=w1139:T3, "Error Out"=w1140:errorcluster)  [unwired: 11 in]
                n88 = call "GEA2MessageFormatter.vi"("Prefix(Send/Recv)"="SEND", "GEA2 Data In"=w1139, "Error In"=w1140) -> ("Output String"=w1141:string, "Error Out"=w1142:errorcluster)  [unwired: 11 in]
                n89 = call "GExplorer_Queue_GEA2.vi"("Output String"=w1141, "error in (no error)"=w1142) -> ("error out"=w1138:errorcluster)  [unwired: 13 in]
                n90 = call "GEA2 Write ERD.vi"("GEA2 Reference In"=w1134, "GEA Inputs"=w1132, "Write ERD List"=w1137, "Error In"=w1138, "Verify ERD Response?"=FALSE) -> ("GEA2 Reference Out"=w1131:refnum<k24>, "Error Out"=w1133:errorcluster)  [unwired: 8 in, 1 out]
              }
              frame "ON" {
                n91 = Concatenate Strings("20" ("string")) -> (w1162:string)
                n92 = Bundle By Name(cluster=w1146, "Data"=w1162) -> (w1161:T25)
                n93 = Build Array(w1161) -> (w1152:T25[])
                n94 = call "Convert Write ERD List to Message.vi"("GEA Inputs"=w1149, "Write ERD List"=w1152, "Error In"=w1150) -> ("GEA Message"=w1154:T3, "Error Out"=w1155:errorcluster)  [unwired: 11 in]
                n95 = call "GEA2MessageFormatter.vi"("Prefix(Send/Recv)"="SEND", "GEA2 Data In"=w1154, "Error In"=w1155) -> ("Output String"=w1156:string, "Error Out"=w1157:errorcluster)  [unwired: 11 in]
                n96 = call "GExplorer_Queue_GEA2.vi"("Output String"=w1156, "error in (no error)"=w1157) -> ("error out"=w1153:errorcluster)  [unwired: 13 in]
                n97 = call "GEA2 Write ERD.vi"("GEA2 Reference In"=w1158, "GEA Inputs"=w1149, "Write ERD List"=w1152, "Error In"=w1153, "Verify ERD Response?"=FALSE) -> ("GEA2 Reference Out"=w1148:refnum<k24>, "Error Out"=w1159:errorcluster)  [unwired: 8 in, 1 out]
              }
            }
          }
          event "Pump.ON", "Pump.OFF": Value Change {
            n98 = event-data() -> ("CtlRef"=w1163:refnum<vi>)  [unwired: 1 in, 5 out]
            n99 = property class="Bool"(reference=w1163, error in=w1166) -> (reference out=w1169:refnum<vi>, error out=w1170:errorcluster, "Label.Text"=w1171:string)
            n100 = Close Reference(reference=w1169, error in (no error)=w1170) -> (error out=w1168:errorcluster)
            n101 = case shown="\"ON\"" w1171 {
              tunnel: [w1176 w1202] -> _
              tunnel: w1165 -> [w1177 w1201]
              tunnel: w1168 -> [w1178 w1193]
              tunnel: w1164 -> [w1175 w1192]
              tunnel: [w1174 w1191] -> _
              tunnel: T25 {"ERD Number"=61441, "Data Type"=enum."string", "Data"=""} ("ERD Read Data In") -> [w1172 w1189]
              frame "OFF", Default {
                n102 = Concatenate Strings("00" ("string")) -> (w1188:string)
                n103 = Bundle By Name(cluster=w1172, "Data"=w1188) -> (w1187:T25)
                n104 = Build Array(w1187) -> (w1180:T25[])
                n105 = call "Convert Write ERD List to Message.vi"("GEA Inputs"=w1175, "Write ERD List"=w1180, "Error In"=w1178) -> ("GEA Message"=w1182:T3, "Error Out"=w1183:errorcluster)  [unwired: 11 in]
                n106 = call "GEA2MessageFormatter.vi"("Prefix(Send/Recv)"="SEND", "GEA2 Data In"=w1182, "Error In"=w1183) -> ("Output String"=w1184:string, "Error Out"=w1185:errorcluster)  [unwired: 11 in]
                n107 = call "GExplorer_Queue_GEA2.vi"("Output String"=w1184, "error in (no error)"=w1185) -> ("error out"=w1181:errorcluster)  [unwired: 13 in]
                n108 = call "GEA2 Write ERD.vi"("GEA2 Reference In"=w1177, "GEA Inputs"=w1175, "Write ERD List"=w1180, "Error In"=w1181, "Verify ERD Response?"=FALSE) -> ("GEA2 Reference Out"=w1174:refnum<k24>, "Error Out"=w1176:errorcluster)  [unwired: 8 in, 1 out]
              }
              frame "ON" {
                n109 = Concatenate Strings("50" ("string")) -> (w1205:string)
                n110 = Bundle By Name(cluster=w1189, "Data"=w1205) -> (w1204:T25)
                n111 = Build Array(w1204) -> (w1195:T25[])
                n112 = call "Convert Write ERD List to Message.vi"("GEA Inputs"=w1192, "Write ERD List"=w1195, "Error In"=w1193) -> ("GEA Message"=w1197:T3, "Error Out"=w1198:errorcluster)  [unwired: 11 in]
                n113 = call "GEA2MessageFormatter.vi"("Prefix(Send/Recv)"="SEND", "GEA2 Data In"=w1197, "Error In"=w1198) -> ("Output String"=w1199:string, "Error Out"=w1200:errorcluster)  [unwired: 11 in]
                n114 = call "GExplorer_Queue_GEA2.vi"("Output String"=w1199, "error in (no error)"=w1200) -> ("error out"=w1196:errorcluster)  [unwired: 13 in]
                n115 = call "GEA2 Write ERD.vi"("GEA2 Reference In"=w1201, "GEA Inputs"=w1192, "Write ERD List"=w1195, "Error In"=w1196, "Verify ERD Response?"=FALSE) -> ("GEA2 Reference Out"=w1191:refnum<k24>, "Error Out"=w1202:errorcluster)  [unwired: 8 in, 1 out]
              }
            }
          }
          event "Main Relay.ON", "Main Relay.OFF": Value Change {
            n116 = event-data() -> ("CtlRef"=w1206:refnum<vi>)  [unwired: 1 in, 5 out]
            n117 = property class="Bool"(reference=w1206, error in=w1209) -> (reference out=w1212:refnum<vi>, error out=w1213:errorcluster, "Label.Text"=w1214:string)
            n118 = Close Reference(reference=w1212, error in (no error)=w1213) -> (error out=w1211:errorcluster)
            n119 = case shown="\"ON\"" w1214 {
              tunnel: [w1219 w1245] -> _
              tunnel: w1208 -> [w1220 w1244]
              tunnel: w1211 -> [w1221 w1236]
              tunnel: w1207 -> [w1218 w1235]
              tunnel: [w1217 w1234] -> _
              tunnel: T25 {"ERD Number"=61441, "Data Type"=enum."string", "Data"=""} ("ERD Read Data In") -> [w1215 w1232]
              frame "OFF", Default {
                n120 = Concatenate Strings("00" ("string")) -> (w1231:string)
                n121 = Bundle By Name(cluster=w1215, "Data"=w1231) -> (w1230:T25)
                n122 = Build Array(w1230) -> (w1223:T25[])
                n123 = call "Convert Write ERD List to Message.vi"("GEA Inputs"=w1218, "Write ERD List"=w1223, "Error In"=w1221) -> ("GEA Message"=w1225:T3, "Error Out"=w1226:errorcluster)  [unwired: 11 in]
                n124 = call "GEA2MessageFormatter.vi"("Prefix(Send/Recv)"="SEND", "GEA2 Data In"=w1225, "Error In"=w1226) -> ("Output String"=w1227:string, "Error Out"=w1228:errorcluster)  [unwired: 11 in]
                n125 = call "GExplorer_Queue_GEA2.vi"("Output String"=w1227, "error in (no error)"=w1228) -> ("error out"=w1224:errorcluster)  [unwired: 13 in]
                n126 = call "GEA2 Write ERD.vi"("GEA2 Reference In"=w1220, "GEA Inputs"=w1218, "Write ERD List"=w1223, "Error In"=w1224, "Verify ERD Response?"=FALSE) -> ("GEA2 Reference Out"=w1217:refnum<k24>, "Error Out"=w1219:errorcluster)  [unwired: 8 in, 1 out]
              }
              frame "ON" {
                n127 = Concatenate Strings("40" ("string")) -> (w1248:string)
                n128 = Bundle By Name(cluster=w1232, "Data"=w1248) -> (w1247:T25)
                n129 = Build Array(w1247) -> (w1238:T25[])
                n130 = call "Convert Write ERD List to Message.vi"("GEA Inputs"=w1235, "Write ERD List"=w1238, "Error In"=w1236) -> ("GEA Message"=w1240:T3, "Error Out"=w1241:errorcluster)  [unwired: 11 in]
                n131 = call "GEA2MessageFormatter.vi"("Prefix(Send/Recv)"="SEND", "GEA2 Data In"=w1240, "Error In"=w1241) -> ("Output String"=w1242:string, "Error Out"=w1243:errorcluster)  [unwired: 11 in]
                n132 = call "GExplorer_Queue_GEA2.vi"("Output String"=w1242, "error in (no error)"=w1243) -> ("error out"=w1239:errorcluster)  [unwired: 13 in]
                n133 = call "GEA2 Write ERD.vi"("GEA2 Reference In"=w1244, "GEA Inputs"=w1235, "Write ERD List"=w1238, "Error In"=w1239, "Verify ERD Response?"=FALSE) -> ("GEA2 Reference Out"=w1234:refnum<k24>, "Error Out"=w1245:errorcluster)  [unwired: 8 in, 1 out]
              }
            }
          }
          event "Buzzer.ON", "Buzzer.OFF": Value Change {
            n134 = event-data() -> ("CtlRef"=w1249:refnum<vi>)  [unwired: 1 in, 5 out]
            n135 = property class="Bool"(reference=w1249, error in=w1252) -> (reference out=w1255:refnum<vi>, error out=w1256:errorcluster, "Label.Text"=w1257:string)
            n136 = Close Reference(reference=w1255, error in (no error)=w1256) -> (error out=w1254:errorcluster)
            n137 = case shown="\"ON\"" w1257 {
              tunnel: [w1262 w1288] -> _
              tunnel: w1251 -> [w1263 w1287]
              tunnel: w1254 -> [w1264 w1279]
              tunnel: w1250 -> [w1261 w1278]
              tunnel: [w1260 w1277] -> _
              tunnel: T25 {"ERD Number"=61442, "Data Type"=enum."string", "Data"=""} ("ERD Read Data In") -> [w1258 w1275]
              frame "OFF", Default {
                n138 = Concatenate Strings("00" ("string")) -> (w1274:string)
                n139 = Bundle By Name(cluster=w1258, "Data"=w1274) -> (w1273:T25)
                n140 = Build Array(w1273) -> (w1266:T25[])
                n141 = call "Convert Write ERD List to Message.vi"("GEA Inputs"=w1261, "Write ERD List"=w1266, "Error In"=w1264) -> ("GEA Message"=w1268:T3, "Error Out"=w1269:errorcluster)  [unwired: 11 in]
                n142 = call "GEA2MessageFormatter.vi"("Prefix(Send/Recv)"="SEND", "GEA2 Data In"=w1268, "Error In"=w1269) -> ("Output String"=w1270:string, "Error Out"=w1271:errorcluster)  [unwired: 11 in]
                n143 = call "GExplorer_Queue_GEA2.vi"("Output String"=w1270, "error in (no error)"=w1271) -> ("error out"=w1267:errorcluster)  [unwired: 13 in]
                n144 = call "GEA2 Write ERD.vi"("GEA2 Reference In"=w1263, "GEA Inputs"=w1261, "Write ERD List"=w1266, "Error In"=w1267, "Verify ERD Response?"=FALSE) -> ("GEA2 Reference Out"=w1260:refnum<k24>, "Error Out"=w1262:errorcluster)  [unwired: 8 in, 1 out]
              }
              frame "ON" {
                n145 = Concatenate Strings("03" ("string")) -> (w1291:string)
                n146 = Bundle By Name(cluster=w1275, "Data"=w1291) -> (w1290:T25)
                n147 = Build Array(w1290) -> (w1281:T25[])
                n148 = call "Convert Write ERD List to Message.vi"("GEA Inputs"=w1278, "Write ERD List"=w1281, "Error In"=w1279) -> ("GEA Message"=w1283:T3, "Error Out"=w1284:errorcluster)  [unwired: 11 in]
                n149 = call "GEA2MessageFormatter.vi"("Prefix(Send/Recv)"="SEND", "GEA2 Data In"=w1283, "Error In"=w1284) -> ("Output String"=w1285:string, "Error Out"=w1286:errorcluster)  [unwired: 11 in]
                n150 = call "GExplorer_Queue_GEA2.vi"("Output String"=w1285, "error in (no error)"=w1286) -> ("error out"=w1282:errorcluster)  [unwired: 13 in]
                n151 = call "GEA2 Write ERD.vi"("GEA2 Reference In"=w1287, "GEA Inputs"=w1278, "Write ERD List"=w1281, "Error In"=w1282, "Verify ERD Response?"=FALSE) -> ("GEA2 Reference Out"=w1277:refnum<k24>, "Error Out"=w1288:errorcluster)  [unwired: 8 in, 1 out]
              }
            }
          }
          event "LEDs.ON", "LEDs.OFF": Value Change {
            n152 = event-data() -> ("CtlRef"=w1292:refnum<vi>)  [unwired: 1 in, 5 out]
            n153 = property class="Bool"(reference=w1292, error in=w1295) -> (reference out=w1298:refnum<vi>, error out=w1299:errorcluster, "Label.Text"=w1300:string)
            n154 = Close Reference(reference=w1298, error in (no error)=w1299) -> (error out=w1297:errorcluster)
            n155 = case shown="\"ON\"" w1300 {
              tunnel: [w1305 w1331] -> _
              tunnel: w1294 -> [w1306 w1330]
              tunnel: w1297 -> [w1307 w1322]
              tunnel: w1293 -> [w1304 w1321]
              tunnel: [w1303 w1320] -> _
              tunnel: T25 {"ERD Number"=61443, "Data Type"=enum."string", "Data"=""} ("ERD Read Data In") -> [w1301 w1318]
              frame "OFF", Default {
                n156 = Concatenate Strings("00" ("string")) -> (w1317:string)
                n157 = Bundle By Name(cluster=w1301, "Data"=w1317) -> (w1316:T25)
                n158 = Build Array(w1316) -> (w1309:T25[])
                n159 = call "Convert Write ERD List to Message.vi"("GEA Inputs"=w1304, "Write ERD List"=w1309, "Error In"=w1307) -> ("GEA Message"=w1311:T3, "Error Out"=w1312:errorcluster)  [unwired: 11 in]
                n160 = call "GEA2MessageFormatter.vi"("Prefix(Send/Recv)"="SEND", "GEA2 Data In"=w1311, "Error In"=w1312) -> ("Output String"=w1313:string, "Error Out"=w1314:errorcluster)  [unwired: 11 in]
                n161 = call "GExplorer_Queue_GEA2.vi"("Output String"=w1313, "error in (no error)"=w1314) -> ("error out"=w1310:errorcluster)  [unwired: 13 in]
                n162 = call "GEA2 Write ERD.vi"("GEA2 Reference In"=w1306, "GEA Inputs"=w1304, "Write ERD List"=w1309, "Error In"=w1310, "Verify ERD Response?"=FALSE) -> ("GEA2 Reference Out"=w1303:refnum<k24>, "Error Out"=w1305:errorcluster)  [unwired: 8 in, 1 out]
              }
              frame "ON" {
                n163 = Concatenate Strings("01" ("string")) -> (w1334:string)
                n164 = Bundle By Name(cluster=w1318, "Data"=w1334) -> (w1333:T25)
                n165 = Build Array(w1333) -> (w1324:T25[])
                n166 = call "Convert Write ERD List to Message.vi"("GEA Inputs"=w1321, "Write ERD List"=w1324, "Error In"=w1322) -> ("GEA Message"=w1326:T3, "Error Out"=w1327:errorcluster)  [unwired: 11 in]
                n167 = call "GEA2MessageFormatter.vi"("Prefix(Send/Recv)"="SEND", "GEA2 Data In"=w1326, "Error In"=w1327) -> ("Output String"=w1328:string, "Error Out"=w1329:errorcluster)  [unwired: 11 in]
                n168 = call "GExplorer_Queue_GEA2.vi"("Output String"=w1328, "error in (no error)"=w1329) -> ("error out"=w1325:errorcluster)  [unwired: 13 in]
                n169 = call "GEA2 Write ERD.vi"("GEA2 Reference In"=w1330, "GEA Inputs"=w1321, "Write ERD List"=w1324, "Error In"=w1325, "Verify ERD Response?"=FALSE) -> ("GEA2 Reference Out"=w1320:refnum<k24>, "Error Out"=w1331:errorcluster)  [unwired: 8 in, 1 out]
              }
            }
          }
          event "Motor.CW", "Motor.OFF", "Motor.CCW": Value Change {
            n170 = event-data() -> ("CtlRef"=w1335:refnum<vi>)  [unwired: 1 in, 5 out]
            n171 = property class="Bool"(reference=w1335, error in=w1338) -> (reference out=w1341:refnum<vi>, error out=w1342:errorcluster, "Label.Text"=w1343:string)
            n172 = Close Reference(reference=w1341, error in (no error)=w1342) -> (error out=w1340:errorcluster)
            n173 = case shown="\"CCW\"" w1343 {
              tunnel: [w1348 w1374 w1391] -> _
              tunnel: w1337 -> [w1349 w1373 w1390]
              tunnel: w1340 -> [w1350 w1365 w1382]
              tunnel: w1336 -> [w1347 w1364 w1381]
              tunnel: [w1346 w1363 w1380] -> _
              tunnel: T25 {"ERD Number"=61441, "Data Type"=enum."string", "Data"=""} ("ERD Read Data In") -> [w1344 w1361 w1378]
              frame "OFF", Default {
                n174 = Concatenate Strings("00" ("string")) -> (w1360:string)
                n175 = Bundle By Name(cluster=w1344, "Data"=w1360) -> (w1359:T25)
                n176 = Build Array(w1359) -> (w1352:T25[])
                n177 = call "Convert Write ERD List to Message.vi"("GEA Inputs"=w1347, "Write ERD List"=w1352, "Error In"=w1350) -> ("GEA Message"=w1354:T3, "Error Out"=w1355:errorcluster)  [unwired: 11 in]
                n178 = call "GEA2MessageFormatter.vi"("Prefix(Send/Recv)"="SEND", "GEA2 Data In"=w1354, "Error In"=w1355) -> ("Output String"=w1356:string, "Error Out"=w1357:errorcluster)  [unwired: 11 in]
                n179 = call "GExplorer_Queue_GEA2.vi"("Output String"=w1356, "error in (no error)"=w1357) -> ("error out"=w1353:errorcluster)  [unwired: 13 in]
                n180 = call "GEA2 Write ERD.vi"("GEA2 Reference In"=w1349, "GEA Inputs"=w1347, "Write ERD List"=w1352, "Error In"=w1353, "Verify ERD Response?"=FALSE) -> ("GEA2 Reference Out"=w1346:refnum<k24>, "Error Out"=w1348:errorcluster)  [unwired: 8 in, 1 out]
              }
              frame "CW" {
                n181 = Concatenate Strings("41" ("string")) -> (w1377:string)
                n182 = Bundle By Name(cluster=w1361, "Data"=w1377) -> (w1376:T25)
                n183 = Build Array(w1376) -> (w1367:T25[])
                n184 = call "Convert Write ERD List to Message.vi"("GEA Inputs"=w1364, "Write ERD List"=w1367, "Error In"=w1365) -> ("GEA Message"=w1369:T3, "Error Out"=w1370:errorcluster)  [unwired: 11 in]
                n185 = call "GEA2MessageFormatter.vi"("Prefix(Send/Recv)"="SEND", "GEA2 Data In"=w1369, "Error In"=w1370) -> ("Output String"=w1371:string, "Error Out"=w1372:errorcluster)  [unwired: 11 in]
                n186 = call "GExplorer_Queue_GEA2.vi"("Output String"=w1371, "error in (no error)"=w1372) -> ("error out"=w1368:errorcluster)  [unwired: 13 in]
                n187 = call "GEA2 Write ERD.vi"("GEA2 Reference In"=w1373, "GEA Inputs"=w1364, "Write ERD List"=w1367, "Error In"=w1368, "Verify ERD Response?"=FALSE) -> ("GEA2 Reference Out"=w1363:refnum<k24>, "Error Out"=w1374:errorcluster)  [unwired: 8 in, 1 out]
              }
              frame "CCW" {
                n188 = Concatenate Strings("42" ("string")) -> (w1394:string)
                n189 = Bundle By Name(cluster=w1378, "Data"=w1394) -> (w1393:T25)
                n190 = Build Array(w1393) -> (w1384:T25[])
                n191 = call "Convert Write ERD List to Message.vi"("GEA Inputs"=w1381, "Write ERD List"=w1384, "Error In"=w1382) -> ("GEA Message"=w1386:T3, "Error Out"=w1387:errorcluster)  [unwired: 11 in]
                n192 = call "GEA2MessageFormatter.vi"("Prefix(Send/Recv)"="SEND", "GEA2 Data In"=w1386, "Error In"=w1387) -> ("Output String"=w1388:string, "Error Out"=w1389:errorcluster)  [unwired: 11 in]
                n193 = call "GExplorer_Queue_GEA2.vi"("Output String"=w1388, "error in (no error)"=w1389) -> ("error out"=w1385:errorcluster)  [unwired: 13 in]
                n194 = call "GEA2 Write ERD.vi"("GEA2 Reference In"=w1390, "GEA Inputs"=w1381, "Write ERD List"=w1384, "Error In"=w1385, "Verify ERD Response?"=FALSE) -> ("GEA2 Reference Out"=w1380:refnum<k24>, "Error Out"=w1391:errorcluster)  [unwired: 8 in, 1 out]
              }
            }
          }
          event "Heaters.Heater 1", "Heaters.BOTH", "Heaters.Heater 2", "Heaters.OFF": Value Change {
            n195 = event-data() -> ("CtlRef"=w1395:refnum<vi>)  [unwired: 1 in, 5 out]
            n196 = property class="Bool"(reference=w1395, error in=w1398) -> (reference out=w1401:refnum<vi>, error out=w1402:errorcluster, "Label.Text"=w1403:string)
            n197 = Close Reference(reference=w1401, error in (no error)=w1402) -> (error out=w1400:errorcluster)
            n198 = case shown="\"Heater 2\"" w1403 {
              tunnel: [w1408 w1434 w1451 w1468] -> _
              tunnel: w1397 -> [w1409 w1433 w1450 w1467]
              tunnel: w1400 -> [w1410 w1425 w1442 w1459]
              tunnel: w1396 -> [w1407 w1424 w1441 w1458]
              tunnel: [w1406 w1423 w1440 w1457] -> _
              tunnel: T25 {"ERD Number"=61441, "Data Type"=enum."string", "Data"=""} ("ERD Read Data In") -> [w1404 w1421 w1438 w1455]
              frame "OFF", Default {
                n199 = Concatenate Strings("00" ("string")) -> (w1420:string)
                n200 = Bundle By Name(cluster=w1404, "Data"=w1420) -> (w1419:T25)
                n201 = Build Array(w1419) -> (w1412:T25[])
                n202 = call "Convert Write ERD List to Message.vi"("GEA Inputs"=w1407, "Write ERD List"=w1412, "Error In"=w1410) -> ("GEA Message"=w1414:T3, "Error Out"=w1415:errorcluster)  [unwired: 11 in]
                n203 = call "GEA2MessageFormatter.vi"("Prefix(Send/Recv)"="SEND", "GEA2 Data In"=w1414, "Error In"=w1415) -> ("Output String"=w1416:string, "Error Out"=w1417:errorcluster)  [unwired: 11 in]
                n204 = call "GExplorer_Queue_GEA2.vi"("Output String"=w1416, "error in (no error)"=w1417) -> ("error out"=w1413:errorcluster)  [unwired: 13 in]
                n205 = call "GEA2 Write ERD.vi"("GEA2 Reference In"=w1409, "GEA Inputs"=w1407, "Write ERD List"=w1412, "Error In"=w1413, "Verify ERD Response?"=FALSE) -> ("GEA2 Reference Out"=w1406:refnum<k24>, "Error Out"=w1408:errorcluster)  [unwired: 8 in, 1 out]
              }
              frame "Heater 1" {
                n206 = Concatenate Strings("45" ("string")) -> (w1437:string)
                n207 = Bundle By Name(cluster=w1421, "Data"=w1437) -> (w1436:T25)
                n208 = Build Array(w1436) -> (w1427:T25[])
                n209 = call "Convert Write ERD List to Message.vi"("GEA Inputs"=w1424, "Write ERD List"=w1427, "Error In"=w1425) -> ("GEA Message"=w1429:T3, "Error Out"=w1430:errorcluster)  [unwired: 11 in]
                n210 = call "GEA2MessageFormatter.vi"("Prefix(Send/Recv)"="SEND", "GEA2 Data In"=w1429, "Error In"=w1430) -> ("Output String"=w1431:string, "Error Out"=w1432:errorcluster)  [unwired: 11 in]
                n211 = call "GExplorer_Queue_GEA2.vi"("Output String"=w1431, "error in (no error)"=w1432) -> ("error out"=w1428:errorcluster)  [unwired: 13 in]
                n212 = call "GEA2 Write ERD.vi"("GEA2 Reference In"=w1433, "GEA Inputs"=w1424, "Write ERD List"=w1427, "Error In"=w1428, "Verify ERD Response?"=FALSE) -> ("GEA2 Reference Out"=w1423:refnum<k24>, "Error Out"=w1434:errorcluster)  [unwired: 8 in, 1 out]
              }
              frame "BOTH" {
                n213 = Concatenate Strings("4D" ("string")) -> (w1454:string)
                n214 = Bundle By Name(cluster=w1438, "Data"=w1454) -> (w1453:T25)
                n215 = Build Array(w1453) -> (w1444:T25[])
                n216 = call "Convert Write ERD List to Message.vi"("GEA Inputs"=w1441, "Write ERD List"=w1444, "Error In"=w1442) -> ("GEA Message"=w1446:T3, "Error Out"=w1447:errorcluster)  [unwired: 11 in]
                n217 = call "GEA2MessageFormatter.vi"("Prefix(Send/Recv)"="SEND", "GEA2 Data In"=w1446, "Error In"=w1447) -> ("Output String"=w1448:string, "Error Out"=w1449:errorcluster)  [unwired: 11 in]
                n218 = call "GExplorer_Queue_GEA2.vi"("Output String"=w1448, "error in (no error)"=w1449) -> ("error out"=w1445:errorcluster)  [unwired: 13 in]
                n219 = call "GEA2 Write ERD.vi"("GEA2 Reference In"=w1450, "GEA Inputs"=w1441, "Write ERD List"=w1444, "Error In"=w1445, "Verify ERD Response?"=FALSE) -> ("GEA2 Reference Out"=w1440:refnum<k24>, "Error Out"=w1451:errorcluster)  [unwired: 8 in, 1 out]
              }
              frame "Heater 2" {
                n220 = Concatenate Strings("49" ("string")) -> (w1471:string)
                n221 = Bundle By Name(cluster=w1455, "Data"=w1471) -> (w1470:T25)
                n222 = Build Array(w1470) -> (w1461:T25[])
                n223 = call "Convert Write ERD List to Message.vi"("GEA Inputs"=w1458, "Write ERD List"=w1461, "Error In"=w1459) -> ("GEA Message"=w1463:T3, "Error Out"=w1464:errorcluster)  [unwired: 11 in]
                n224 = call "GEA2MessageFormatter.vi"("Prefix(Send/Recv)"="SEND", "GEA2 Data In"=w1463, "Error In"=w1464) -> ("Output String"=w1465:string, "Error Out"=w1466:errorcluster)  [unwired: 11 in]
                n225 = call "GExplorer_Queue_GEA2.vi"("Output String"=w1465, "error in (no error)"=w1466) -> ("error out"=w1462:errorcluster)  [unwired: 13 in]
                n226 = call "GEA2 Write ERD.vi"("GEA2 Reference In"=w1467, "GEA Inputs"=w1458, "Write ERD List"=w1461, "Error In"=w1462, "Verify ERD Response?"=FALSE) -> ("GEA2 Reference Out"=w1457:refnum<k24>, "Error Out"=w1468:errorcluster)  [unwired: 8 in, 1 out]
              }
            }
          }
          event "Test Mode.Exit", "Test Mode.Enter": Value Change {
            n227 = event-data() -> ("CtlRef"=w1472:refnum<vi>)  [unwired: 1 in, 5 out]
            n228 = property class="Bool"(reference=w1472, error in=w1475) -> (reference out=w1478:refnum<vi>, error out=w1479:errorcluster, "Label.Text"=w1480:string)
            n229 = Close Reference(reference=w1478, error in (no error)=w1479) -> (error out=w1477:errorcluster)
            n230 = case shown="\"Exit\"" w1480 {
              tunnel: [w1485 w1511] -> _
              tunnel: w1474 -> [w1486 w1510]
              tunnel: w1477 -> [w1487 w1502]
              tunnel: w1473 -> [w1484 w1501]
              tunnel: [w1483 w1500] -> _
              tunnel: T25 {"ERD Number"=61440, "Data Type"=enum."string", "Data"=""} ("ERD Read Data In") -> [w1481 w1498]
              frame "Enter", Default {
                n231 = Concatenate Strings("01" ("string")) -> (w1497:string)
                n232 = Bundle By Name(cluster=w1481, "Data"=w1497) -> (w1496:T25)
                n233 = Build Array(w1496) -> (w1489:T25[])
                n234 = call "Convert Write ERD List to Message.vi"("GEA Inputs"=w1484, "Write ERD List"=w1489, "Error In"=w1487) -> ("GEA Message"=w1491:T3, "Error Out"=w1492:errorcluster)  [unwired: 11 in]
                n235 = call "GEA2MessageFormatter.vi"("Prefix(Send/Recv)"="SEND", "GEA2 Data In"=w1491, "Error In"=w1492) -> ("Output String"=w1493:string, "Error Out"=w1494:errorcluster)  [unwired: 11 in]
                n236 = call "GExplorer_Queue_GEA2.vi"("Output String"=w1493, "error in (no error)"=w1494) -> ("error out"=w1490:errorcluster)  [unwired: 13 in]
                n237 = call "GEA2 Write ERD.vi"("GEA2 Reference In"=w1486, "GEA Inputs"=w1484, "Write ERD List"=w1489, "Error In"=w1490, "Verify ERD Response?"=FALSE) -> ("GEA2 Reference Out"=w1483:refnum<k24>, "Error Out"=w1485:errorcluster)  [unwired: 8 in, 1 out]
              }
              frame "Exit" {
                n238 = Concatenate Strings("00" ("string")) -> (w1514:string)
                n239 = Bundle By Name(cluster=w1498, "Data"=w1514) -> (w1513:T25)
                n240 = Build Array(w1513) -> (w1504:T25[])
                n241 = call "Convert Write ERD List to Message.vi"("GEA Inputs"=w1501, "Write ERD List"=w1504, "Error In"=w1502) -> ("GEA Message"=w1506:T3, "Error Out"=w1507:errorcluster)  [unwired: 11 in]
                n242 = call "GEA2MessageFormatter.vi"("Prefix(Send/Recv)"="SEND", "GEA2 Data In"=w1506, "Error In"=w1507) -> ("Output String"=w1508:string, "Error Out"=w1509:errorcluster)  [unwired: 11 in]
                n243 = call "GExplorer_Queue_GEA2.vi"("Output String"=w1508, "error in (no error)"=w1509) -> ("error out"=w1505:errorcluster)  [unwired: 13 in]
                n244 = call "GEA2 Write ERD.vi"("GEA2 Reference In"=w1510, "GEA Inputs"=w1501, "Write ERD List"=w1504, "Error In"=w1505, "Verify ERD Response?"=FALSE) -> ("GEA2 Reference Out"=w1500:refnum<k24>, "Error Out"=w1511:errorcluster)  [unwired: 8 in, 1 out]
              }
            }
          }
          event "Clear Fault Table Buffer": Value Change {
            n245 = event-data() -> ()  [unwired: 1 in, 6 out]
            n246 = Bundle By Name(cluster=T25 {"ERD Number"=130, "Data Type"=enum."string", "Data"=""} ("ERD Read Data In"), "Data"="FF") -> (w1530:T25)
            n247 = Build Array(w1530) -> (w1524:T25[])
            n248 = call "Convert Write ERD List to Message.vi"("GEA Inputs"=w1521, "Write ERD List"=w1524, "Error In"=w1520) -> ("GEA Message"=w1526:T3, "Error Out"=w1527:errorcluster)  [unwired: 11 in]
            n249 = call "GEA2MessageFormatter.vi"("Prefix(Send/Recv)"="SEND", "GEA2 Data In"=w1526, "Error In"=w1527) -> ("Output String"=w1528:string, "Error Out"=w1529:errorcluster)  [unwired: 11 in]
            n250 = call "GExplorer_Queue_GEA2.vi"("Output String"=w1528, "error in (no error)"=w1529) -> ("error out"=w1525:errorcluster)  [unwired: 13 in]
            n251 = call "GEA2 Write ERD.vi"("GEA2 Reference In"=w1519, "Read Timeout (ms)"=u32 2000, "GEA Inputs"=w1521, "Write ERD List"=w1524, "Error In"=w1525, "Verify ERD Response?"=FALSE) -> ("GEA2 Reference Out"=w1518:refnum<k24>, "Error Out"=w1517:errorcluster)  [unwired: 7 in, 1 out]
          }
          event "Clear Cycle Buffer": Value Change {
            n252 = event-data() -> ()  [unwired: 1 in, 6 out]
            n253 = Build Array(T25 {"ERD Number"=136, "Data Type"=enum."string", "Data"="FF"} ("ERD Read Data In")) -> (w1544:T25[])
            n254 = call "Convert Write ERD List to Message.vi"("GEA Inputs"=w1539, "Write ERD List"=w1544, "Error In"=w1542) -> ("GEA Message"=w1546:T3, "Error Out"=w1547:errorcluster)  [unwired: 11 in]
            n255 = call "GEA2MessageFormatter.vi"("Prefix(Send/Recv)"="SEND", "GEA2 Data In"=w1546, "Error In"=w1547) -> ("Output String"=w1548:string, "Error Out"=w1549:errorcluster)  [unwired: 11 in]
            n256 = call "GExplorer_Queue_GEA2.vi"("Output String"=w1548, "error in (no error)"=w1549) -> ("error out"=w1545:errorcluster)  [unwired: 13 in]
            n257 = call "GEA2 Write ERD.vi"("GEA2 Reference In"=w1541, "GEA Inputs"=w1539, "Write ERD List"=w1544, "Error In"=w1545) -> ("Error Out"=w1538:errorcluster)  [unwired: 9 in, 2 out]
            n258 = call "Time Delay6"("error in (no error)"=w1538) -> ("error out"=w1533:errorcluster)  [unwired: 10 in]
            n259 = property on="Get Cycle History" class="Bool (strict)"(error in=w1533, "Val(Sgnl)"=TRUE ("Get Cycle History")) -> (error out=w1537:errorcluster)  [unwired: 1 in, 1 out]
            n260 = call "Time Delay7"("error in (no error)"=w1537) -> ("error out"=w1532:errorcluster)  [unwired: 10 in]
            n261 = property on="Get Cycle History" class="Bool (strict)"(error in=w1532, "Val(Sgnl)"=FALSE ("Get Cycle History")) -> (error out=w1536:errorcluster)  [unwired: 1 in, 1 out]
          }
          event "Get Cycle History": Value Change {
            w1556 = T6[] [{"ERD Number"=135, "Data Type"=enum."string"}, {"ERD Number"=57344, "Data Type"=enum."string"}, {"ERD Number"=57345, "Data Type"=enum."string"}, {"ERD Number"=57346, "Data Type"=enum."string"}, {"ERD Number"=57347, "Data Type"=enum."string"}, {"ERD Number"=57348, "Data Type"=enum."string"}, {"ERD Number"=57349, "Data Type"=enum."string"}, {"ERD Number"=57350, "Data Type"=enum."string"}, {"ERD Number"=57351, "Data Type"=enum."string"}, {"ERD Number"=57352, "Data Type"=enum."string"}, {"ERD Number"=57353, "Data Type"=enum."string"}] ("Read ERD List")
            n262 = event-data() -> ()  [unwired: 1 in, 6 out]
            n263 = call "Convert Read ERD List to Message.vi"("GEA Inputs"=w1551, "Read ERD List"=w1556, "Error In"=w1558) -> ("GEA Message"=w1562:T3, "Error Out"=w1563:errorcluster)  [unwired: 11 in]
            n264 = call "GEA2MessageFormatter.vi"("Prefix(Send/Recv)"="SEND", "GEA2 Data In"=w1562, "Error In"=w1563) -> ("Output String"=w1561:string, "Error Out"=w1560:errorcluster)  [unwired: 11 in]
            n265 = call "GExplorer_Queue_GEA2.vi"("Output String"=w1561, "error in (no error)"=w1560) -> ("error out"=w1557:errorcluster)  [unwired: 13 in]
            n266 = call "GEA2 Read ERD Multiple Messages.vi"("GEA2 Reference In"=w1552, "Read Timeout (ms)"=u32 500, "GEA Inputs"=w1551, "Read ERD List"=w1556, "Error In"=w1557, "#ERDs per message"=4, "Verify ERD Response?"=TRUE) -> ("ERD Data Out"=w1564:T31[], "Error Out"=w1555:errorcluster)  [unwired: 5 in, 2 out]
            n267 = call "Cycle_Diag_Table_Read_FL24_Dryer.vi"("ERD Data In"=w1564, "error in (no error)"=w1555) -> ("Cycle Buffer Status"=→"Cycle Buffer Status":T14, "Diag Cycle String Out"=→"Diagnostics Table":string[][], "error out"=w1550:errorcluster)  [unwired: 11 in]
          }
          event "Save Cycle History Log": Value Change {
            w1572 = T6[] [{"ERD Number"=135, "Data Type"=enum."string"}, {"ERD Number"=57344, "Data Type"=enum."string"}, {"ERD Number"=57345, "Data Type"=enum."string"}, {"ERD Number"=57346, "Data Type"=enum."string"}, {"ERD Number"=57347, "Data Type"=enum."string"}, {"ERD Number"=57348, "Data Type"=enum."string"}, {"ERD Number"=57349, "Data Type"=enum."string"}, {"ERD Number"=57350, "Data Type"=enum."string"}, {"ERD Number"=57351, "Data Type"=enum."string"}, {"ERD Number"=57352, "Data Type"=enum."string"}, {"ERD Number"=57353, "Data Type"=enum."string"}] ("Read ERD List")
            n268 = event-data() -> ()  [unwired: 1 in, 6 out]
            n269 = call "Convert Read ERD List to Message.vi"("GEA Inputs"=w1575, "Read ERD List"=w1572, "Error In"=w1574) -> ("GEA Message"=w1581:T3, "Error Out"=w1582:errorcluster)  [unwired: 11 in]
            n270 = call "GEA2MessageFormatter.vi"("Prefix(Send/Recv)"="SEND", "GEA2 Data In"=w1581, "Error In"=w1582) -> ("Output String"=w1580:string, "Error Out"=w1579:errorcluster)  [unwired: 11 in]
            n271 = call "GExplorer_Queue_GEA2.vi"("Output String"=w1580, "error in (no error)"=w1579) -> ("error out"=w1577:errorcluster)  [unwired: 13 in]
            n272 = call "GEA2 Read ERD Multiple Messages.vi"("GEA2 Reference In"=w1573, "Read Timeout (ms)"=u32 500, "GEA Inputs"=w1575, "Read ERD List"=w1572, "Error In"=w1577, "#ERDs per message"=4, "Verify ERD Response?"=TRUE) -> ("ERD Data Out"=w1571:T31[], "Error Out"=w1576:errorcluster)  [unwired: 5 in, 2 out]
            n273 = call "Cycle_Diag_Table_Read_FL24_Dryer.vi"("ERD Data In"=w1571, "error in (no error)"=w1576) -> ("Diag Cycle String Out"=w1570:string[][], "error out"=w1569:errorcluster)  [unwired: 11 in, 1 out]
            n274 = call "Cycle_History_Logging.vi"("error in (no error)"=w1569, "Diag Cycle String Out"=w1570) -> ("error out"=w1568:errorcluster)  [unwired: 9 in]
          }
          event "Data ON": Value Change {
            n275 = event-data() -> ()  [unwired: 1 in, 6 out]
            n276 = case shown="True" "Data ON" {
              tunnel: w1589 -> [w1592 w1596]
              tunnel: [w1591 w1595] -> w1588
              tunnel: w1586 -> [w1590 w1594]
              frame True {
                n277 = Enqueue Element(queue=w1590, element=T22 {"Data"=variant, "State"=enum."Init"} ("Data"), error in (no error)=w1592) -> (error out=w1591:errorcluster)  [unwired: 1 in, 2 out]
              }
              frame False {
                n278 = Enqueue Element(queue=w1594, element=T22 {"Data"=variant, "State"=enum."Pause"} ("Data"), error in (no error)=w1596) -> (error out=w1595:errorcluster)  [unwired: 1 in, 2 out]
              }
            }
          }
          event "Stop": Value Change; User Event; Panel Close {
            n279 = event-data() -> ()  [unwired: 1 in, 3 out]
            n280 = call "Control_ERD_Loop_Brass.vi"("Command (ERD Loop Control)"=ERD_Loop_Control_Command_Brass."Shutdown", "Error In"=w1606) -> ("Error Out"=w1605:errorcluster)  [unwired: 13 in]
            n281 = call "Control_GEA2_Loop_Brass.vi"("Command (ERD Loop Control)"=GEA2_Control_Command_Brass."Shutdown", "Error In"=w1605) -> ("Error Out"=w1607:errorcluster)  [unwired: 13 in]
            n282 = call "Control_DAQ_Loop_Brass.vi"("Command (DAQ Control)"=DAQ_Control_Command_Brass."Shutdown", "Error In"=w1607) -> ("Error Out"=w1610:errorcluster)  [unwired: 13 in]
            n283 = call "Control_Cont_Send_Brass.vi"("Command (ERD Loop Control)"=GEA2_Control_Command_Brass."Shutdown", "Error In"=w1610) -> ("Error Out"=w1600:errorcluster)  [unwired: 13 in]
            n284 = call "Time Delay8"("error in (no error)"=w1600, "Delay Time (s)"=2.0) -> ("error out"=w1599:errorcluster)  [unwired: 9 in]
          }
        }
        n285 = call "Error_Control_Brass.vi"("Error In"=w1012) -> ("Error Out"=w1014:errorcluster)  [unwired: 14 in]
      }
      n286 = Unbundle By Name(T22 {"Data"=variant, "State"=enum."Init"} ("Data")) -> ("State"=w68:T23)
      n287 = Build Array(w22, w63, w61, w62) -> (w60:refnum<vi>[])
      n288 = while "DAQ Loop" {
        shift-right: [w487] -> w95
        shift-left: w32 -> [w485]
        shift-right: [w464] -> _
        shift-left: DAQ_States_Brass."Wait for Init" ("States") -> [w482]
        shift-right: [w465] -> _
        shift-left: "Wait for Init" ("Report Text") -> [w480]
        tunnel: w59 -> [w481]
        shift-right: [w463] -> _
        shift-left: _ -> [w420]
        shift-right: [w462] -> _
        shift-left: FALSE -> [w461]
        shift-right: [w451] -> _
        shift-left: w51 -> [w450]
        shift-right: [w449] -> _
        shift-left: w51 -> [w448]
        shift-right: [w447] -> _
        shift-left: w51 -> [w446]
        shift-right: [w445] -> _
        shift-left: w51 -> [w444]
        shift-right: [w443] -> _
        shift-left: w51 -> [w442]
        shift-right: [w441] -> _
        shift-left: w51 -> [w440]
        shift-right: [w439] -> _
        shift-left: w51 -> [w438]
        shift-right: [w425] -> _
        shift-left: 1.0 -> [w421]
        shift-right: [w424] -> _
        shift-left: 1.0 -> [w428]
        shift-right: [w423] -> _
        shift-left: 0.0 -> [w427]
        shift-right: [w419] -> _
        shift-left: w51 -> [w418]
        shift-right: [w417] -> _
        shift-left: FALSE -> [w452]
        stop <- w477 stop-if-true
        # "Automatic Modeshift Feedback"
        # "DAQ Loop"
        n289 = Greater?(x=w428, y=5.0 ("x")) -> (0:w430:bool)
        n290 = Dequeue Element(queue=w481, timeout in ms (-1)=0, error in (no error)=w485) -> (element=w483:T21, timed out?=w484:bool, error out=w476:errorcluster)  [unwired: 1 out]
        n291 = Wait (ms)(milliseconds to wait=u32 250) -> ()  [unwired: 1 out]
        n292 = Select(t="Basket RPM", s=w430, f=w421) -> (s? t:f=w425:dbl)
        n293 = Select(t=w482, s=w484, f=w483) -> (s? t:f=w479:T21)
        n294 = Multiply(x=w425, y=0.40625) -> (x*y=w456:dbl)
        n295 = Less?(x=w425, y=1.0) -> (x < y?=w454:bool)
        n296 = Equal?(x=w421, y=w425) -> (x = y?=w453:bool)
        n297 = case shown="\"Run\"" w479 {
          selector: w479 -> [_ _ _ _ _ _ w966]
          tunnel: [_ _ _ w679 w799 _ _] -> w419
          tunnel: [w519 w543 w575 w680 w797 w904 w969] -> w473
          tunnel: w438 -> [w534 w558 w583 _ w796 w898 w915]
          tunnel: [w534 w558 w583 w684 w795 _ _] -> w439
          tunnel: w440 -> [w533 w557 w584 _ w794 w895 w942]
          tunnel: [w533 w557 w584 w688 w793 _ _] -> w441
          tunnel: [w517 w541 w567 w687 w792 w858 w932] -> w471
          tunnel: [w518 w542 w568 w683 w791 w865 w944] -> w472
          tunnel: [w528 DAQ_States_Brass."Verify Hardware" ("t") w580 DAQ_States_Brass."Run" ("t") w769 DAQ_States_Brass."Wait for Init" ("States") w966] -> w464
          tunnel: [FALSE FALSE FALSE TRUE TRUE FALSE FALSE] -> w463
          tunnel: w446 -> [w532 w556 w587 _ w754 w902 w971]
          tunnel: [w514 w538 w564 w676 w788 w851 w929] -> w468
          tunnel: [w532 w556 w587 w677 w789 _ _] -> w447
          tunnel: [w515 w539 w565 w640 w779 w890 w970] -> w469
          tunnel: w444 -> [w531 w555 w586 _ w778 w901 w965]
          tunnel: [w531 w555 w586 w645 w780 _ _] -> w445
          tunnel: [_ _ _ _ _ FALSE TRUE] -> w477
          tunnel: [_ _ _ _ w787 _ _] -> w437
          tunnel: [_ _ _ _ w781 _ _] -> w422
          tunnel: [_ _ _ _ w786 _ _] -> w436
          tunnel: [_ _ _ _ w785 _ _] -> w435
          tunnel: [_ _ _ _ w784 _ _] -> w434
          tunnel: [_ _ _ _ w783 _ _] -> w433
          tunnel: [_ _ _ _ w782 _ _] -> w432
          tunnel: [w516 w540 w566 w637 w777 w888 w963] -> w470
          tunnel: [w530 w554 w585 w634 w775 _ _] -> w443
          tunnel: w442 -> [w530 w554 w585 _ w776 w889 w964]
          tunnel: [_ _ _ _ w774 _ _] -> w460
          tunnel: [_ _ _ _ w773 _ _] -> w459
          tunnel: [w529 w553 w577 "Initialize" ("Report Text") "Running" ("Report Text") "Wait for Init" ("Report Text") "Exit" ("Report Text")] -> w465
          tunnel: w480 -> [w529 w553 _ _ _ _ _]
          tunnel: [w513 w537 w563 w618 w761 w882 w960] -> w467
          tunnel: [w524 w551 w573 w615 w760 _ _] -> w449
          tunnel: [w523 w550 w572 w613 w758 _ _] -> w451
          tunnel: [w512 w536 w562 w612 w759 w881 w907] -> w466
          tunnel: w448 -> [w524 w551 w573 _ w762 w883 w961]
          tunnel: w450 -> [w523 w550 w572 _ w757 w879 w927]
          tunnel: [w511 w535 w561 w592 w756 FALSE FALSE] -> w462
          tunnel: [FALSE FALSE FALSE FALSE w746 FALSE FALSE] -> w417
          tunnel: [w520 w546 w570 w599 w745 w874 w957] -> w474
          tunnel: "Turn On DAQ" -> [w521 _ _ _ w721 _ _]
          tunnel: w476 -> [w519 w543 w569 w601 w744 w873 w956]
          tunnel: w476 -> [w518 w542 w568 w600 w739 w871 w918]
          tunnel: w476 -> [w520 w545 w570 w599 w745 w874 w957]
          tunnel: w476 -> [w517 w541 w567 w598 w737 w856 w941]
          tunnel: w476 -> [w516 w540 w566 w597 w736 w855 w955]
          tunnel: w476 -> [w515 w539 w565 w596 w733 w854 w954]
          tunnel: w476 -> [w514 w538 w564 w595 w732 w853 w953]
          tunnel: w476 -> [w513 w537 w563 w594 w726 w849 w952]
          tunnel: w476 -> [w512 w536 w562 w593 w722 w848 w926]
          tunnel: w461 -> [w511 w535 w561 w592 w725 _ _]
          tunnel: w456 -> [_ _ _ _ w731 _ _]
          tunnel: 0.5 ("Duty Cycle") -> [_ _ _ _ w730 _ _]
          tunnel: w454 -> [_ _ _ _ w728 _ _]
          tunnel: w453 -> [_ _ _ _ w729 _ _]
          tunnel: w452 -> [_ _ _ _ w727 _ _]
          tunnel: w420 -> [_ _ _ _ _ _ w951]
          tunnel: w418 -> [_ _ _ _ w720 w847 w950]
          frame "Wait for Init", Default {
            # "Hall Sensor"
            # "Motor TRIAC CCW"
            # "Motor TRIAC CW"
            # "Relay Controls"
            # "TRIAC Outputs"
            # "AO for ADC"
            n298 = Select(t=DAQ_States_Brass."Rename Devices", s=w521, f=DAQ_States_Brass."Wait for Init" ("States")) -> (s? t:f=w528:T21)
          }
          frame "Rename Devices" {
            # "Hall Sensor"
            # "Motor TRIAC CCW"
            # "Motor TRIAC CW"
            # "Relay Controls"
            # "TRIAC Outputs"
            n299 = case shown="\"LE\"" "HE/LE ?" {
              tunnel: ["VALEW_HE" "VALEW_LE"] -> w547
              frame "HE", Default {
              }
              frame "LE" {
              }
            }
            n300 = call "VALEW_Rename DAQmx Devices.vi"("cDAQ Name"=w547, "Error In"=w545) -> ("Error Out"=w546:errorcluster)  [unwired: 13 in]
          }
          frame "Verify Hardware" {
            n301 = call "DeviceListCheck.vi"("Device List"=string[] ["9481_1", "9435_1", "9435_2", "9401_1", "9269_1"], "Error In"=w569) -> ("Devices Present?"=w574:bool, "Report Text"=w577:string, "Error Out"=w576:errorcluster)  [unwired: 11 in]
            n302 = case shown="False" w574 {
              selector: w574 -> [w589 _]
              tunnel: w576 -> [w590 w591]
              tunnel: [w588 w591] -> w575
              frame False {
                n303 = property on="Turn On DAQ" class="Bool (strict)"(error in=w590, "Value"=w589) -> (error out=w588:errorcluster)  [unwired: 1 in, 1 out]
              }
              frame True {
              }
            }
            n304 = Select(t=DAQ_States_Brass."Initialize" ("f"), s=w574, f=DAQ_States_Brass."Wait for Init") -> (s? t:f=w580:T21)
          }
          frame "Initialize" {
            w606 = 4 items=["verify"=2, "reserve"=4, "commit"=3, "unreserve"=5, "abort"=6] ("action")
            w622 = 10123 items=["Finite Samples"=10178, "Continuous Samples"=10123, "Hardware Timed Single Point"=12522] ("sample mode")
            w625 = 4 items=["verify"=2, "reserve"=4, "commit"=3, "unreserve"=5, "abort"=6] ("action")
            w658 = 4 items=["verify"=2, "reserve"=4, "commit"=3, "unreserve"=5, "abort"=6] ("action")
            w659 = 4 items=["verify"=2, "reserve"=4, "commit"=3, "unreserve"=5, "abort"=6] ("action")
            w673 = 10123 items=["Finite Samples"=10178, "Continuous Samples"=10123, "Hardware Timed Single Point"=12522] ("sample mode")
            w681 = 0 items=["one channel for each line", "one channel for all lines"] ("line grouping")
            w686 = 0 items=["one channel for each line", "one channel for all lines"] ("line grouping")
            w689 = 0.0  # minimum value
            w690 = 5.0  # maximum value
            # "Hall Sensor"
            # "Motor TRIAC CCW"
            # "Motor TRIAC CW"
            # "Relay Controls"
            # "TRIAC Outputs"
            # "AO for ADC"
            n305 = call <vilib>:"DAQmx Create Task.vi"("auto cleanup"=TRUE, "error in"=w595) -> ("task out"=w647:refnum<k21>, "error out"=w648:errorcluster)  [unwired: 12 in]
            n306 = call <vilib>:"DAQmx Create Task.vi"("auto cleanup"=TRUE, "error in"=w594) -> ("task out"=w621:refnum<k21>, "error out"=w620:errorcluster)  [unwired: 12 in]
            n307 = call <vilib>:"DAQmx Create Task.vi"("auto cleanup"=TRUE, "error in"=w597) -> ("task out"=w655:refnum<k21>, "error out"=w656:errorcluster)  [unwired: 12 in]
            n308 = call <vilib>:"DAQmx Create Task.vi"("auto cleanup"=TRUE, "error in"=w596) -> ("task out"=w653:refnum<k21>, "error out"=w654:errorcluster)  [unwired: 12 in]
            n309 = call-poly <vilib>:"DAQmx Create Virtual Channel.vi"("task in"=w647, "counter"=tag "9401_1/ctr2", "error in"=w648) -> ("task out"=w650:refnum<k21>, "error out"=w678:errorcluster)  [unwired: 11 in]
            n310 = call-poly <vilib>:"DAQmx Create Virtual Channel.vi"("task in"=w655, "counter"=tag "9401_1/ctr0", "error in"=w656) -> ("task out"=w668:refnum<k21>, "error out"=w664:errorcluster)  [unwired: 11 in]
            n311 = call-poly <vilib>:"DAQmx Create Virtual Channel.vi"("task in"=w653, "counter"=tag "9401_1/ctr1", "error in"=w654) -> ("task out"=w667:refnum<k21>, "error out"=w666:errorcluster)  [unwired: 11 in]
            n312 = call-poly <vilib>:"DAQmx Create Virtual Channel.vi"("task in"=w621, "lines"=tag "9401_1/port0/line2", "error in"=w620) -> ("task out"=w627:refnum<k21>, "error out"=w628:errorcluster)  [unwired: 11 in]
            n313 = property class="DAQmx Channel"(reference=w650, error in=w678, "CO.Pulse.Term"=tag "/9401_1/PFI4") -> (reference out=w675:refnum<k21>, error out=w674:errorcluster)
            n314 = call-poly <vilib>:"DAQmx Create Virtual Channel.vi"("lines"=tag "9481_1/port0/line3", "error in"=w593) -> ("task out"=w613:refnum<k21>, "error out"=w612:errorcluster)  [unwired: 12 in]
            n315 = property class="DAQmx Channel"(reference=w668, error in=w664, "CI.CountEdges.Term"=tag "/9401_1/PFI0") -> (reference out=w663:refnum<k21>, error out=w662:errorcluster)
            n316 = property class="DAQmx Channel"(reference=w667, error in=w666, "CI.CountEdges.Term"=tag "/9401_1/PFI1") -> (reference out=w661:refnum<k21>, error out=w660:errorcluster)
            n317 = call-poly <vilib>:"DAQmx Create Virtual Channel.vi"("lines"=tag "9481_1/port0/line0:2", "name to assign"="Relay Outputs", "line grouping"=w686, "error in"=w600) -> ("task out"=w684:refnum<k21>, "error out"=w683:errorcluster)  [unwired: 10 in]
            n318 = call-poly <vilib>:"DAQmx Create Virtual Channel.vi"("lines"=tag "9435_1/port0/line0:2, 9435_2/port0/line0:3", "name to assign"="Outputs", "line grouping"=w681, "error in"=w601) -> ("task out"=w679:refnum<k21>, "error out"=w680:errorcluster)  [unwired: 10 in]
            n319 = call-poly <vilib>:"DAQmx Create Virtual Channel.vi"("maximum value"=w690, "minimum value"=w689, "physical channels"=tag "9269_1/ao0:2" ("lines"), "name to assign"="AO for ADC", "error in"=w598) -> ("task out"=w688:refnum<k21>, "error out"=w687:errorcluster)  [unwired: 9 in]
            n320 = call-poly <vilib>:"DAQmx Timing.vi"("task/channels in"=w627, "sample mode"=w622, "rate"=1000.0, "error in"=w628) -> ("task out"=w623:refnum<k21>, "error out"=w624:errorcluster)  [unwired: 10 in]
            n321 = call-poly <vilib>:"DAQmx Timing.vi"("task/channels in"=w675, "sample mode"=w673, "error in"=w674) -> ("task out"=w605:refnum<k21>, "error out"=w602:errorcluster)  [unwired: 11 in]
            n322 = call <vilib>:"DAQmx Control Task.vi"("task/channels in"=w663, "action"=w658, "error in"=w662) -> ("task out"=w636:refnum<k21>, "error out"=w639:errorcluster)  [unwired: 11 in]
            n323 = call <vilib>:"DAQmx Control Task.vi"("task/channels in"=w661, "action"=w659, "error in"=w660) -> ("task out"=w644:refnum<k21>, "error out"=w642:errorcluster)  [unwired: 11 in]
            n324 = call <vilib>:"DAQmx Control Task.vi"("task/channels in"=w605, "action"=w606, "error in"=w602) -> ("task out"=w604:refnum<k21>, "error out"=w603:errorcluster)  [unwired: 11 in]
            n325 = call <vilib>:"DAQmx Control Task.vi"("task/channels in"=w623, "action"=w625, "error in"=w624) -> ("task out"=w616:refnum<k21>, "error out"=w617:errorcluster)  [unwired: 11 in]
            n326 = flat-sequence {
              tunnel: w604 -> [w694]
              tunnel: w603 -> [w693]
              tunnel: w644 -> [w702]
              tunnel: [w702] -> w643
              tunnel: w642 -> [w701]
              tunnel: [w701] -> w641
              tunnel: w639 -> [w700]
              tunnel: [w700] -> w638
              tunnel: w636 -> [w699]
              tunnel: [w699] -> w635
              tunnel: w617 -> [w697]
              tunnel: w616 -> [w698]
              tunnel: [w696] -> w610
              tunnel: [w695] -> w609
              tunnel: [w694] -> w608
              tunnel: [w693] -> w607
              tunnel: [w706] -> w676
              tunnel: [w705] -> w677
              tunnel: [w716] -> w645
              tunnel: w643 -> [w715]
              tunnel: w641 -> [w714]
              tunnel: [w713] -> w640
              tunnel: w638 -> [w712]
              tunnel: [w711] -> w637
              tunnel: w635 -> [w710]
              tunnel: [w709] -> w634
              tunnel: [w708] -> w618
              tunnel: [w707] -> w615
              tunnel: w610 -> [w708]
              tunnel: w609 -> [w707]
              tunnel: w608 -> [w704]
              tunnel: w607 -> [w703]
              frame #0 {
                n327 = call <vilib>:"DAQmx Start Task.vi"("task/channels in"=w698, "error in"=w697) -> ("task out"=w695:refnum<k21>, "error out"=w696:errorcluster)  [unwired: 12 in]
              }
              frame #1 {
                n328 = call <vilib>:"DAQmx Start Task.vi"("task/channels in"=w710, "error in"=w712) -> ("task out"=w709:refnum<k21>, "error out"=w711:errorcluster)  [unwired: 12 in]
                n329 = call <vilib>:"DAQmx Start Task.vi"("task/channels in"=w715, "error in"=w714) -> ("task out"=w716:refnum<k21>, "error out"=w713:errorcluster)  [unwired: 12 in]
                n330 = call <vilib>:"DAQmx Start Task.vi"("task/channels in"=w704, "error in"=w703) -> ("task out"=w705:refnum<k21>, "error out"=w706:errorcluster)  [unwired: 12 in]
              }
            }
          }
          frame "Run" {
            # "Lid Lock Feedback"
            # "Is the task stopped?"
            # "Hall Sensor"
            # "Motor TRIAC CCW"
            # "Motor TRIAC CW"
            # "AO for ADC"
            # "Relay Controls"
            # "TRIAC Outputs"
            n331 = case shown="True" w728 {
              tunnel: w754 -> [w833 w838]
              tunnel: [w833 w837] -> w752
              tunnel: [w832 w836] -> w753
              tunnel: [w831 TRUE] -> w747
              tunnel: w732 -> [w832 w834]
              tunnel: w727 -> [w831 _]
              frame False {
              }
              frame True {
                n332 = call <vilib>:"DAQmx Stop Task.vi"("task/channels in"=w838, "error in"=w834) -> ("task out"=w837:refnum<k21>, "error out"=w836:errorcluster)  [unwired: 12 in]
              }
            }
            n333 = call-poly <vilib>:"DAQmx Read.vi"("task/channels in"=w762, "number of samples per channel"=-1, "timeout"=10.0, "error in"=w726) -> ("task out"=w760:refnum<k21>, "data"=w766:u8[], "error out"=w761:errorcluster)  [unwired: 9 in]
            n334 = Compound Arithmetic op=AND(w747, invert w728) -> (w749:bool)
            n335 = case shown="False" w749 {
              tunnel: w753 -> [w823 w827]
              tunnel: w752 -> [w824 w826]
              tunnel: [w824 w830] -> w751
              tunnel: [w823 w829] -> w750
              tunnel: w747 -> [w822 _]
              tunnel: [w822 FALSE] -> w746
              frame False {
              }
              frame True {
                n336 = call <vilib>:"DAQmx Start Task.vi"("task/channels in"=w826, "error in"=w827) -> ("task out"=w830:refnum<k21>, "error out"=w829:errorcluster)  [unwired: 12 in]
                n337 = Wait (ms)(milliseconds to wait=u32 1200) -> ()  [unwired: 1 out]
              }
            }
            n338 = Build Array("AC Power", "Mode Shift FB", "Lid Status") -> (w740:bool[])
            n339 = Build Array("Pressure", "Motor Current", "Temperature") -> (w738:dbl[])
            n340 = Search 1D Array(1D array=w766, element=u8 4) -> (index of element=w764:i32)  [unwired: 1 in]
            n341 = Equal?(x=w764, y=-1) -> (x = y?=w755:bool)
            n342 = Compound Arithmetic op=OR(w728, w729) -> (w748:bool)
            n343 = call-poly <vilib>:"DAQmx Read.vi"("task/channels in"=w720, "error in"=w744) -> ("task out"=w799:refnum<k21>, "data"=w798:bool[], "error out"=w797:errorcluster)  [unwired: 11 in]
            n344 = call-poly <vilib>:"DAQmx Write.vi"("task/channels in"=w796, "data"=w740, "error in"=w739) -> ("task out"=w795:refnum<k21>, "error out"=w791:errorcluster)  [unwired: 10 in, 1 out]
            n345 = call-poly <vilib>:"DAQmx Write.vi"("task/channels in"=w794, "data"=w738, "error in"=w737) -> ("task out"=w793:refnum<k21>, "error out"=w792:errorcluster)  [unwired: 10 in, 1 out]
            n346 = call-poly <vilib>:"DAQmx Read.vi"("task/channels in"=w776, "error in"=w736) -> ("task out"=w775:refnum<k21>, "data"=w735:u32, "error out"=w777:errorcluster)  [unwired: 11 in]
            "CW" <- w735
            n347 = call-poly <vilib>:"DAQmx Read.vi"("task/channels in"=w778, "error in"=w733) -> ("task out"=w780:refnum<k21>, "data"=w734:u32, "error out"=w779:errorcluster)  [unwired: 11 in]
            "CCW" <- w734
            n348 = case shown="True" "LL (M - A)" {
              tunnel: [w802 w812] -> w759
              tunnel: [w803 w811] -> w758
              tunnel: w757 -> [w805 w810]
              tunnel: [w801 w809] -> w756
              tunnel: w755 -> [_ w808]
              tunnel: "Lid Lock Feedback" -> [w804 _]
              tunnel: w725 -> [w801 w807]
              tunnel: w722 -> [w800 w806]
              frame False {
                n349 = call-poly <vilib>:"DAQmx Write.vi"("task/channels in"=w805, "data"=w804, "error in"=w800) -> ("task out"=w803:refnum<k21>, "error out"=w802:errorcluster)  [unwired: 10 in, 1 out]
              }
              frame True {
                # "Automatic Lid Lock feedback"
                n350 = case shown="True" w808 {
                  tunnel: w810 -> [w818 w821]
                  tunnel: [w817 w820] -> w812
                  tunnel: [w816 w821] -> w811
                  tunnel: [w815 w819] -> w809
                  tunnel: w807 -> [w814 w819]
                  tunnel: w806 -> [w813 w820]
                  frame False {
                    n351 = Not(x=w814) -> (.not. x?=w815:bool)
                    n352 = call-poly <vilib>:"DAQmx Write.vi"("task/channels in"=w818, "data"=w815, "error in"=w813) -> ("task out"=w816:refnum<k21>, "error out"=w817:errorcluster)  [unwired: 10 in, 1 out]
                  }
                  frame True {
                  }
                }
              }
            }
            n353 = Index Array(array=w798) -> (element #1=w787:bool, element #2=w781:bool, element #3=w786:bool, element #4=w785:bool, element #5=w784:bool, element #6=w783:bool, element #7=w782:bool)  [unwired: 7 in]
            n354 = call "Counts to Triac Direction.vi"("CCW ctr"=w734, "CW ctr"=w735) -> ("CW"=w773:bool, "CCW"=w774:bool)  [unwired: 8 in]
            n355 = case shown="False" w748 {
              tunnel: w751 -> [w844 w846]
              tunnel: w750 -> [w843 w845]
              tunnel: [w842 w846] -> w789
              tunnel: [w841 w845] -> w788
              tunnel: w731 -> [w840 _]
              tunnel: w730 -> [w839 _]
              frame False {
                n356 = property class="DAQmx Channel"(reference=w844, error in=w843, "CO.Pulse.Freq"=w840, "CO.Pulse.DutyCyc"=w839) -> (reference out=w842:refnum<k21>, error out=w841:errorcluster)
              }
              frame True {
              }
            }
            n357 = Select(t=DAQ_States_Brass."Run" ("States"), s=w721, f=DAQ_States_Brass."Shutdown" ("States")) -> (s? t:f=w769:T21)
          }
          frame "Shutdown" {
            w887 = 0.0
            w884 = FALSE ("element")
            # "Hall Sensor"
            # "Motor TRIAC CCW"
            # "Motor TRIAC CW"
            # "Relay Controls"
            # "TRIAC Outputs"
            # "AO for ADC"
            n358 = local read "AC Power"() -> (w872:bool)
            n359 = Build Array(w872, w884, w884) -> (w899:bool[])
            n360 = Build Array(w887, w887, w887) -> (w886:dbl[])
            n361 = call-poly <vilib>:"DAQmx Write.vi"("task/channels in"=w898, "data"=w899, "error in"=w871) -> ("task out"=w892:refnum<k21>, "error out"=w893:errorcluster)  [unwired: 10 in, 1 out]
            n362 = call-poly <vilib>:"DAQmx Write.vi"("task/channels in"=w879, "data"=FALSE, "error in"=w848) -> ("task out"=w878:refnum<k21>, "error out"=w877:errorcluster)  [unwired: 10 in, 1 out]
            n363 = call-poly <vilib>:"DAQmx Write.vi"("task/channels in"=w895, "data"=w886, "error in"=w856) -> ("task out"=w897:refnum<k21>, "error out"=w896:errorcluster)  [unwired: 10 in, 1 out]
            n364 = call "Time Delay4"("error in (no error)"=w893, "Delay Time (s)"=2.0) -> ("error out"=w891:errorcluster)  [unwired: 9 in]
            n365 = call <vilib>:"DAQmx Clear Task.vi"("task in"=w883, "error in"=w849) -> ("error out"=w882:errorcluster)  [unwired: 13 in]
            n366 = call <vilib>:"DAQmx Clear Task.vi"("task in"=w847, "error in"=w873) -> ("error out"=w904:errorcluster)  [unwired: 13 in]
            n367 = call <vilib>:"DAQmx Clear Task.vi"("task in"=w892, "error in"=w891) -> ("error out"=w870:errorcluster)  [unwired: 13 in]
            n368 = call <vilib>:"DAQmx Clear Task.vi"("task in"=w897, "error in"=w896) -> ("error out"=w863:errorcluster)  [unwired: 13 in]
            n369 = call <vilib>:"DAQmx Clear Task.vi"("task in"=w889, "error in"=w855) -> ("error out"=w888:errorcluster)  [unwired: 13 in]
            n370 = call <vilib>:"DAQmx Clear Task.vi"("task in"=w901, "error in"=w854) -> ("error out"=w890:errorcluster)  [unwired: 13 in]
            n371 = call <vilib>:"DAQmx Clear Task.vi"("task in"=w902, "error in"=w853) -> ("error out"=w852:errorcluster)  [unwired: 13 in]
            n372 = call <vilib>:"DAQmx Clear Task.vi"("task in"=w878, "error in"=w877) -> ("error out"=w881:errorcluster)  [unwired: 13 in]
            n373 = property on="Motor Current" class="Slide (strict)"(error in=w863, "Value"=2.5 ("Motor Current")) -> (error out=w861:errorcluster)  [unwired: 1 in, 1 out]
            n374 = property on="Turn On DAQ" class="Bool (strict)"(error in=w870, "Value"=FALSE ("Turn On DAQ")) -> (error out=w868:errorcluster)  [unwired: 1 in, 1 out]
            n375 = property on="Basket RPM" class="DigNum (strict)"(error in=w852, "Value"=1.0 ("Basket RPM")) -> (error out=w851:errorcluster)  [unwired: 1 in, 1 out]
            n376 = property on="Temperature" class="Slide (strict)"(error in=w861, "Value"=2.5 ("Temperature")) -> (error out=w859:errorcluster)  [unwired: 1 in, 1 out]
            n377 = property on="Mode Shift FB" class="Bool (strict)"(error in=w868, "Value"=FALSE ("Mode Shift FB")) -> (error out=w866:errorcluster)  [unwired: 1 in, 1 out]
            n378 = property on="Lid Status" class="Bool (strict)"(error in=w866, "Value"=FALSE ("Lid Status")) -> (error out=w865:errorcluster)  [unwired: 1 in, 1 out]
            n379 = property on="Pressure" class="Slide (strict)"(error in=w859, "Value"=0.0 ("Pressure")) -> (error out=w858:errorcluster)  [unwired: 1 in, 1 out]
          }
          frame "Exit" {
            w922 = FALSE ("element")
            w940 = 0.0
            n380 = local read "AC Power"() -> (w923:bool)
            n381 = Build Array(w923, w922, w922) -> (w919:bool[])
            n382 = call-poly <vilib>:"DAQmx Write.vi"("task/channels in"=w915, "data"=w919, "error in"=w918) -> ("task out"=w916:refnum<k21>, "error out"=w921:errorcluster)  [unwired: 10 in, 1 out]
            n383 = Build Array(w940, w940, w940) -> (w943:dbl[])
            n384 = call-poly <vilib>:"DAQmx Write.vi"("task/channels in"=w927, "data"=FALSE, "error in"=w926) -> ("task out"=w925:refnum<k21>, "error out"=w924:errorcluster)  [unwired: 10 in, 1 out]
            n385 = call-poly <vilib>:"DAQmx Write.vi"("task/channels in"=w942, "data"=w943, "error in"=w941) -> ("task out"=w939:refnum<k21>, "error out"=w938:errorcluster)  [unwired: 10 in, 1 out]
            n386 = call "Time Delay"("error in (no error)"=w921, "Delay Time (s)"=2.0) -> ("error out"=w917:errorcluster)  [unwired: 9 in]
            n387 = case shown="True" w951 {
              tunnel: w916 -> [_ w1003]
              tunnel: w971 -> [_ w1002]
              tunnel: [w975 w1001] -> w930
              tunnel: [w976 w1000] -> w970
              tunnel: [w972 w999] -> w910
              tunnel: [w978 w998] -> w913
              tunnel: [w979 w997] -> w969
              tunnel: w965 -> [_ w996]
              tunnel: w964 -> [_ w995]
              tunnel: [w977 w994] -> w963
              tunnel: w961 -> [_ w993]
              tunnel: [w974 w992] -> w960
              tunnel: w925 -> [_ w991]
              tunnel: [w973 w990] -> w908
              tunnel: w956 -> [w979 w989]
              tunnel: w917 -> [w978 w988]
              tunnel: w955 -> [w977 w987]
              tunnel: w954 -> [w976 w986]
              tunnel: w953 -> [w975 w985]
              tunnel: w952 -> [w974 w984]
              tunnel: w924 -> [w973 w983]
              tunnel: w950 -> [_ w982]
              tunnel: w939 -> [_ w981]
              tunnel: w938 -> [w972 w980]
              frame False {
              }
              frame True {
                # "Hall Sensor"
                # "Motor TRIAC CCW"
                # "Motor TRIAC CW"
                # "Relay Controls"
                # "TRIAC Outputs"
                # "AO for ADC"
                n388 = call <vilib>:"DAQmx Clear Task.vi"("task in"=w993, "error in"=w984) -> ("error out"=w992:errorcluster)  [unwired: 13 in]
                n389 = call <vilib>:"DAQmx Clear Task.vi"("task in"=w991, "error in"=w983) -> ("error out"=w990:errorcluster)  [unwired: 13 in]
                n390 = call <vilib>:"DAQmx Clear Task.vi"("task in"=w982, "error in"=w989) -> ("error out"=w997:errorcluster)  [unwired: 13 in]
                n391 = call <vilib>:"DAQmx Clear Task.vi"("task in"=w1003, "error in"=w988) -> ("error out"=w998:errorcluster)  [unwired: 13 in]
                n392 = call <vilib>:"DAQmx Clear Task.vi"("task in"=w981, "error in"=w980) -> ("error out"=w999:errorcluster)  [unwired: 13 in]
                n393 = call <vilib>:"DAQmx Clear Task.vi"("task in"=w995, "error in"=w987) -> ("error out"=w994:errorcluster)  [unwired: 13 in]
                n394 = call <vilib>:"DAQmx Clear Task.vi"("task in"=w996, "error in"=w986) -> ("error out"=w1000:errorcluster)  [unwired: 13 in]
                n395 = call <vilib>:"DAQmx Clear Task.vi"("task in"=w1002, "error in"=w985) -> ("error out"=w1001:errorcluster)  [unwired: 13 in]
              }
            }
            n396 = call <vilib>:"Clear Errors.vi"("error in (no error)"=w910, "specific error code to clear (0: all)"=-200088) -> ("error out"=w909:errorcluster)  [unwired: 4 in, 1 out]
            n397 = call <vilib>:"Clear Errors.vi"("error in (no error)"=w913, "specific error code to clear (0: all)"=-200088) -> ("error out"=w912:errorcluster)  [unwired: 4 in, 1 out]
            n398 = call <vilib>:"Clear Errors.vi"("error in (no error)"=w908, "specific error code to clear (0: all)"=-200088) -> ("error out"=w907:errorcluster)  [unwired: 4 in, 1 out]
            n399 = property on="Turn On DAQ" class="Bool (strict)"(error in=w912, "Value"=FALSE ("Turn On DAQ")) -> (error out=w948:errorcluster)  [unwired: 1 in, 1 out]
            n400 = property on="Motor Current" class="Slide (strict)"(error in=w909, "Value"=2.5 ("Motor Current")) -> (error out=w936:errorcluster)  [unwired: 1 in, 1 out]
            n401 = property on="Basket RPM" class="DigNum (strict)"(error in=w930, "Value"=1.0 ("Basket RPM")) -> (error out=w929:errorcluster)  [unwired: 1 in, 1 out]
            n402 = property on="Mode Shift FB" class="Bool (strict)"(error in=w948, "Value"=FALSE ("Mode Shift FB")) -> (error out=w946:errorcluster)  [unwired: 1 in, 1 out]
            n403 = property on="Temperature" class="Slide (strict)"(error in=w936, "Value"=2.5 ("Temperature")) -> (error out=w934:errorcluster)  [unwired: 1 in, 1 out]
            n404 = property on="Lid Status" class="Bool (strict)"(error in=w946, "Value"=FALSE ("Lid Status")) -> (error out=w944:errorcluster)  [unwired: 1 in, 1 out]
            n405 = property on="Pressure" class="Slide (strict)"(error in=w934, "Value"=0.0 ("Pressure")) -> (error out=w932:errorcluster)  [unwired: 1 in, 1 out]
          }
        }
        "DAQ Status" <- w465
        "DAQ On?" <- w463
        "Triac CW" <- w460
        "Traic CCW" <- w459
        "Cold Valve" <- w435
        "Recirc Pump" <- w436
        "Mode Shift" <- w422
        "Drain Pump" <- w437
        "Fabric SoftValve" <- w432
        "Spray/Rinse Valve" <- w433
        "Hot Valve" <- w434
        n406 = case shown="True" "MS (M - A)" {
          tunnel: w427 -> [w489 w500]
          tunnel: [w489 w499] -> w423
          tunnel: w422 -> [_ w490]
          frame False {
          }
          frame True {
            n407 = Equal?(x=w490, y=TRUE) -> (x = y?=w497:bool)
            n408 = case shown="True" w497 {
              tunnel: w500 -> [w505 w507]
              tunnel: [w505 w506] -> w492
              frame False {
              }
              frame True {
                n409 = Increment(x=w507) -> (x+1=w506:dbl)
              }
            }
            n410 = In Range and Coerce(upper limit=24.0, x=w492, lower limit=15.0) -> (In Range?=w494:bool)  [unwired: 1 out]
            n411 = case shown="True" w494 {
              frame False {
                n412 = property on="Mode Shift FB" class="Bool (strict)"("Value"=FALSE ("Mode Shift FB")) -> ()  [unwired: 2 in, 2 out]
              }
              frame True {
                n413 = property on="Mode Shift FB" class="Bool (strict)"("Value"=TRUE ("Mode Shift FB")) -> ()  [unwired: 2 in, 2 out]
              }
            }
            n414 = Greater Or Equal?(x=w492, y=24.0) -> (x >= y?=w491:bool)
            n415 = case shown="True" w491 {
              tunnel: w492 -> [w501 _]
              tunnel: [w501 0.0] -> w499
              frame False {
              }
              frame True {
              }
            }
          }
        }
        n416 = case shown="False" w430 {
          tunnel: w428 -> [w509 _]
          tunnel: [w508 0.0] -> w424
          frame False {
            n417 = Increment(x=w509) -> (x+1=w508:dbl)
          }
          frame True {
          }
        }
        n418 = Merge Errors(w474, w473, w472, w471, w470, w469, w468, w467, w466) -> (w475:errorcluster)
        n419 = call "Error_Control_Brass.vi"("Error In"=w475) -> ("Error Out"=w487:errorcluster)  [unwired: 14 in]
      }
      n420 = while "Periodic ERD Query Loop" {
        shift-right: [w187] -> w49
        shift-left: w76 -> [w189]
        tunnel: w66 -> [w190]
        shift-right: [w184] -> _
        shift-left: _ -> [w183]
        shift-right: [w178] -> _
        shift-left: w68 -> [w180]
        shift-right: [w173] -> _
        shift-left: _ -> [w172]
        tunnel: w64 -> [w171]
        tunnel: [w170] -> w47
        shift-right: [w169] -> _
        shift-left: _ -> [w168]
        tunnel: w60 -> [w167]
        i -> [w166]
        stop <- w186 stop-if-true
        # "ERD Loop"
        n421 = Dequeue Element(queue=w190, timeout in ms (-1)=0, error in (no error)=w189) -> (element=w175:T22, timed out?=w181:bool, error out=w188:errorcluster)  [unwired: 1 out]
        n422 = Unbundle By Name(w175) -> ("State"=w165:T23)
        n423 = Select(t=w180, s=w181, f=w165) -> (s? t:f=w179:T23)
        n424 = call "FGV_GEA2_Ref.vi"("Action"=enum16{"Set Ref", "Get Ref"}."Get Ref", "Error In"=w188) -> ("GEA2 Reference Out"=w174:refnum<k24>, "Error Out"=w177:errorcluster)  [unwired: 12 in]
        n425 = case shown="\"Update Graphs\"" w179 {
          tunnel: w177 -> [w200 w208 w221 w235 w255 w292 w339 w367 w375]
          tunnel: [w192 w204 w214 w235 w253 w291 w336 w367 w375] -> w185
          tunnel: [_ _ _ _ _ _ _ _ TRUE] -> w186
          tunnel: [w199 w206 w212 w238 w259 w285 w346 w368 w373] -> w184
          tunnel: w183 -> [w199 w206 w233 w238 w259 w285 w346 w368 w373]
          tunnel: T5 {"Source"=229, "Destination"=53} ("GEA Inputs") -> [_ _ w210 _ w243 w289 _ _ _]
          tunnel: [ERD_Loop_States_Brass."Build ERD Read List" ("State") ERD_Loop_States_Brass."Read ERDs" ("State") ERD_Loop_States_Brass."Update UI" ("State") ERD_Loop_States_Brass."Update Graphs" ("State") ERD_Loop_States_Brass."Read Faults" ("State") ERD_Loop_States_Brass."Log Data" ("State") ERD_Loop_States_Brass."Read ERDs" ("State") ERD_Loop_States_Brass."Pause" ("State") ERD_Loop_States_Brass."Shutdown" ("State")] -> w178
          tunnel: w174 -> [_ _ w222 _ w248 w290 _ _ _]
          tunnel: [w197 w207 w211 w240 w257 w286 w345 w365 w371] -> w173
          tunnel: w172 -> [w197 _ w211 w240 w257 w286 w345 w365 w371]
          tunnel: w171 -> [w196 w203 w219 w236 w256 w284 w344 w364 w370]
          tunnel: [w196 w203 w219 w236 w256 w284 w343 w364 w370] -> w170
          tunnel: [w195 w202 w213 w237 w247 w287 w322 w363 w369] -> w169
          tunnel: w168 -> [w195 w202 _ w237 w245 w288 w322 w363 w369]
          tunnel: w167 -> [_ _ _ _ w249 _ _ _ _]
          tunnel: w166 -> [_ _ _ _ _ _ _ _ _]
          frame "Init", Default {
            # "Set Write Header\nFGV to True"
            n426 = call "Write_Header_FGV.vi"("Write Header ? In"=TRUE, "Action"=enum16{"Get", "Set"}."Set", "Error In"=w200) -> ("Error Out"=w192:errorcluster)  [unwired: 11 in, 1 out]
          }
          frame "Build ERD Read List" {
            n427 = call "ERD_Read_List_Builder.vi"("Array"="ERD Read List", "Error In"=w208) -> ("Read ERD List"=w207:T6[], "Error Out"=w204:errorcluster)  [unwired: 16 in]
          }
          frame "Read ERDs" {
            n428 = call "Convert Read ERD List to Message.vi"("GEA Inputs"=w210, "Read ERD List"=w211, "Error In"=w221) -> ("GEA Message"=w230:T3, "Error Out"=w231:errorcluster)  [unwired: 11 in]
            n429 = call "GEA2MessageFormatter.vi"("Prefix(Send/Recv)"="SEND", "GEA2 Data In"=w230, "Error In"=w231) -> ("Output String"=w229:string, "Error Out"=w228:errorcluster)  [unwired: 11 in]
            n430 = call "GExplorer_Queue_GEA2.vi"("Output String"=w229, "error in (no error)"=w228) -> ("error out"=w226:errorcluster)  [unwired: 13 in]
            n431 = Tick Count (ms)() -> (millisecond timer value=w212:u32)
            n432 = Subtract(x=w212, y=w233) -> (x-y=→"Log Rate (ms)":u32)
            n433 = call "GEA2 Read ERD Multiple Messages.vi"("GEA2 Reference In"=w222, "Retry Count"=1, "Read Timeout (ms)"=u32 250, "GEA Inputs"=w210, "Read ERD List"=w211, "Error In"=w226, "#ERDs per message"=5, "Verify ERD Response?"=FALSE) -> ("ERD Data Out"=w209:T31[], "Error Out"=w218:errorcluster)  [unwired: 4 in, 2 out]
            n434 = call "Write_Header_FGV.vi"("Action"=enum16{"Get", "Set"}."Get", "Error In"=w218) -> ("Write Header ? Out"=w215:bool, "Error Out"=w217:errorcluster)  [unwired: 12 in]
            n435 = call "Convert_ERDs_Brass.vi"("New Header?"=w215, "Array"=w209, "Error In"=w217) -> ("All_ERD_Data_Bundled_Brass"=w213:T32, "Error Out"=w214:errorcluster)  [unwired: 11 in]
          }
          frame "Update UI" {
            n436 = Unbundle By Name(w237) -> ("Version"=→"Version":T4, "ERD_Always Show"=→"ERD_Always Show":T1)
          }
          frame "Update Graphs" {
            n437 = case shown="True" "ERD Graphing ON" {
              tunnel: w255 -> [w273 w281]
              tunnel: [w273 w280] -> w254
              tunnel: "ERD Graph Cntrl" -> [_ w279]
              tunnel: [_ w278] -> w250
              tunnel: w248 -> [_ w277]
              tunnel: w245 -> [w272 w276]
              tunnel: [w272 w275] -> w244
              tunnel: w243 -> [_ w274]
              frame False {
              }
              frame True {
                n438 = call "Graph ERD Read List_Brass.vi"("GEA2 Reference In"=w277, "GEA Inputs"=w274, "All_Bundled_Data_Brass"=w276, "ERD Graph Cntrl"=w279, "Error In"=w281) -> ("ERD Graph  Ind"=w278:T10, "All_Bundled_Data_Brass 2"=w275:T32, "Error Out"=w280:errorcluster)  [unwired: 7 in, 1 out]
              }
            }
            n439 = case shown="True" "Graphing ON" {
              tunnel: w254 -> [w260 w271]
              tunnel: [w260 w270] -> w253
              tunnel: w250 -> [_ w268]
              tunnel: w249 -> [_ w264]
              tunnel: w244 -> [w261 w263]
              tunnel: [w261 w263] -> w247
              frame False {
              }
              frame True {
                n440 = call "Update Graphs_Brass.vi"("Select Graph"="Select Graph", "appended array"=w264, "ERD Graph  Ind 2"=w268, "All_Bundled_Data_Brass"=w263, "Error In"=w271) -> ("All Loads"=→"All Loads":u16[][], "ERD 3"=→"ERD 3":dbl, "ERD 2"=→"ERD 2":dbl, "ERD 1"=→"ERD 1":dbl, "Error Out"=w270:errorcluster)  [unwired: 6 in]
                "ERD Graph  Ind" <- w268
              }
            }
          }
          frame "Read Faults" {
            n441 = case shown="True" "Fault ON" {
              tunnel: w292 -> [w293 w302]
              tunnel: [w293 w301] -> w291
              tunnel: w290 -> [_ w300]
              tunnel: w289 -> [_ w299]
              tunnel: w288 -> [w294 w298]
              tunnel: [w294 w297] -> w287
              frame False {
              }
              frame True {
                # "0-9 Sequence\n10-20 Table"
                n442 = call "GEA2 Read ERD Multiple Messages.vi"("GEA2 Reference In"=w300, "Retry Count"=2, "Read Timeout (ms)"=u32 250 ("Read Timeout (ms) 2"), "GEA Inputs"=w299, "Read ERD List"=T6[] [{"ERD Number"=132, "Data Type"=enum."string"}, {"ERD Number"=141, "Data Type"=enum."uint32_t"}, {"ERD Number"=57374, "Data Type"=enum."string"}, {"ERD Number"=57375, "Data Type"=enum."string"}, {"ERD Number"=57376, "Data Type"=enum."string"}, {"ERD Number"=57377, "Data Type"=enum."string"}, {"ERD Number"=57378, "Data Type"=enum."string"}, {"ERD Number"=57379, "Data Type"=enum."string"}, {"ERD Number"=57380, "Data Type"=enum."string"}, {"ERD Number"=57381, "Data Type"=enum."string"}, {"ERD Number"=129, "Data Type"=enum."string"}, {"ERD Number"=57474, "Data Type"=enum."string"}, {"ERD Number"=57475, "Data Type"=enum."string"}, {"ERD Number"=57476, "Data Type"=enum."string"}, {"ERD Number"=57477, "Data Type"=enum."string"}, {"ERD Number"=57478, "Data Type"=enum."string"}, {"ERD Number"=57479, "Data Type"=enum."string"}, {"ERD Number"=57480, "Data Type"=enum."string"}, {"ERD Number"=57481, "Data Type"=enum."string"}, {"ERD Number"=57482, "Data Type"=enum."string"}, {"ERD Number"=57483, "Data Type"=enum."string"}], "Error In"=w302, "#ERDs per message"=5 ("#ERDs per message 2"), "Verify ERD Response?"=FALSE) -> ("ERD Data Out"=w307:T31[], "Error Out"=w301:errorcluster)  [unwired: 4 in, 2 out]
                n443 = Array Subset(array=w307, index=10, length=11) -> (w308:T31[])
                n444 = Array Subset(array=w307, index=0, length=10) -> (w306:T31[])
                n445 = call "Fault_Table_Read.vi"("ERD Data Out"=w308) -> ("Fault Set?"=→"Fault Status":bool, "Table Buffer Status"=→"Table Buffer Status":T13, "Fault Table String Out"=→"Fault Table Buffer":string[][], "Fault Table Array Out"=w296:T34)  [unwired: 11 in]
                n446 = call "Fault_Seq_Read.vi"("Seq ERD In"=w306) -> ("Seq Buffer Status"=→"Seq Buffer Status":T13, "String"=→"Fault Sequence Buffer":string)  [unwired: 13 in]
                n447 = Bundle By Name(cluster=w298, "Fault Table Array"=w296) -> (w297:T32)
              }
            }
          }
          frame "Log Data" {
            # "TimeStamp"
            # "Append With Fault Log Data"
            # "Write Date/Time Header"
            n448 = Unbundle By Name(w322) -> ("CSV File String Arrays.ERD Name Array"=w342:string[], "CSV File String Arrays.ERD Number Array"=w341:string[], "CSV File String Arrays.ERD Converted String Data"=w334:string[])
            n449 = call "Write_Header_FGV.vi"("Action"=enum16{"Get", "Set"}."Get", "Error In"=w339) -> ("Write Header ? Out"=w320:bool, "Error Out"=w333:errorcluster)  [unwired: 12 in]
            n450 = case shown="True" w320 {
              tunnel: w342 -> [w355 _]
              tunnel: [w357 string[] [] ("ERD Name Array")] -> w332
              tunnel: w341 -> [w356 _]
              tunnel: [w360 string[] [] ("ERD Number Array")] -> w330
              frame True {
                n451 = Insert Into Array(array=w356, index=0, new element #1="", new element #2="", new element #3="", new element #4="") -> (w360:string[])
                n452 = Insert Into Array(array=w355, index=0, new element #1="Date", new element #2="Time", new element #3="HH:MM:SS", new element #4=".SS" ("new element/subarray")) -> (w357:string[])
              }
              frame False {
              }
            }
            n453 = call "TimeStamp to String Array.vi"("String Array In"=w334) -> ("String Array Out"=w328:string[])  [unwired: 10 in]
            n454 = Unbundle By Name(w322) -> ("Fault Table Array"=w321:T34)
            n455 = call "Faults_To_String_Array.vi"("Write Header ?"=w320, "Fault Table Entry"=w321, "Error In"=w333) -> ("Fault Header String Array"=w327:string[], "Fault ERD Number String Array"=w326:string[], "Fault Data String Array"=w325:string[], "Error Out"=w323:errorcluster)  [unwired: 13 in]
            n456 = Insert Into Array(array=w332, new element=w327) -> (w331:string[])  [unwired: 1 in]
            n457 = Insert Into Array(array=w330, new element=w326) -> (w329:string[])  [unwired: 1 in]
            n458 = Insert Into Array(array=w328, new element=w325) -> (w324:string[])  [unwired: 1 in]
            n459 = call "Write _To_CSV_File.vi"("Refnum In"=w344, "String Array 1"=w331, "String Array 2"=w329, "String Array 3"=w324, "Error In"=w323) -> ("Refnum Out"=w343:refnum<file>, "Error Out"=w337:errorcluster)  [unwired: 12 in, 1 out]
            n460 = call "Write_Header_FGV.vi"("Write Header ? In"=FALSE, "Action"=enum16{"Get", "Set"}."Set", "Error In"=w337) -> ("Error Out"=w336:errorcluster)  [unwired: 11 in, 1 out]
          }
          frame "Pause" {
          }
          frame "Shutdown" {
          }
        }
        n461 = call "Error_Control_Brass.vi"("Error In"=w185) -> ("Error Out"=w187:errorcluster)  [unwired: 14 in]
      }
      n462 = while "GEA2 Receive Message Loop" {
        shift-right: [w1614] -> w126
        shift-left: w32 -> [w1615]
        shift-right: [w1611] -> _
        shift-left: w115 -> [w1616]
        stop <- w1613 stop-if-true
        # "GEA2 Receive Message Loop"
        n463 = event shown="[0] <Data>: User Event" {
          selector: w1616 -> [w1632 w1634 w1650 w1656]
          dyn-events: [w1632 w1634 w1645 w1656] -> w1611
          timeout: _ -> [_ _ _ _]
          tunnel: w1615 -> [w1631 w1636 w1653 w1658]
          tunnel: [w1619 w1636 w1638 w1658] -> w1612
          tunnel: [FALSE TRUE _ TRUE] -> w1613
          event User Event {
            n464 = event-data() -> ("Source"=w1626:u8, "Destination"=w1625:u8, "Command"=w1624:u8, "Message"=w1623:string)  [unwired: 1 in]
            n465 = Bundle By Name(cluster=T3 {"Source"=0, "Destination"=0, "Command"=0, "Message"=""} ("GEA2 Msg"), "Source"=w1626, "Destination"=w1625, "Command"=w1624, "Message"=w1623) -> (w1617:T3)
            n466 = call "GEA2 Log Filter.vi"("Filter Log"="Filter Log", "Filter Data"="Filter Data", "GEA2 Msg"=w1617, "Cmd to Filter"="Cmd", "error in (no error)"=w1631) -> ("error out"=w1620:errorcluster)  [unwired: 10 in]
            n467 = call "FGV_GEA2_Ref.vi"("Action"=enum16{"Set Ref", "Get Ref"}."Get Ref", "Error In"=w1620) -> ("GEA2 Reference Out"=w1618:refnum<k24>, "Error Out"=w1621:errorcluster)  [unwired: 12 in]
            n468 = call "ACK Subscriptions Publications.vi"("GEA2 Reference In"=w1618, "GEA2 Msg"=w1617, "error in (no error)"=w1621) -> ("error out"=w1619:errorcluster)  [unwired: 11 in, 1 out]
          }
          event User Event {
            n469 = event-data() -> ()  [unwired: 1 in, 1 out]
          }
          event "Board Index": Value Change {
            # "Stop old GEA2\nbus reference"
            # "Allow other references a chance\nto begin using new reference"
            # "Store new GEA2 bus reference"
            # "Update event registration\nand initialize new GEA2 bus"
            # "Get the previous GEA2\nbus ref, but don't stop it\nuntil we update the FGV\nwith the new GEA2 ref"
            n470 = event-data() -> ("NewVal"=w1649:u8)  [unwired: 1 in]
            n471 = property on="Board Index" class="DigNum (strict)"(error in=w1653, "DisabledEnum"=T29."Disabled and Grayed Out" ("Disabled")) -> (error out=w1654:errorcluster)  [unwired: 1 in, 1 out]
            n472 = call "FGV_GEA2_Ref.vi"("Action"=enum16{"Set Ref", "Get Ref"}."Get Ref", "Error In"=w1654) -> ("GEA2 Reference Out"=w1637:refnum<k24>, "Error Out"=w1651:errorcluster)  [unwired: 12 in]
            n473 = call "GEA2_Reregister.vi"("Board Index"=w1649, "Event Registration In"=w1650, "Error In"=w1651) -> ("GEA2 Reference Out"=w1643:refnum<k24>, "Board ID"=w1646:string, "Event Registration Out"=w1645:refnum<event-registration>, "Error Out"=w1647:errorcluster)  [unwired: 9 in]
            n474 = property on="Board Index" class="DigNum (strict)"(error in=w1647, "DisabledEnum"=T29."Enabled" ("Disabled")) -> (error out=w1644:errorcluster)  [unwired: 1 in, 1 out]
            n475 = local write "Board ID"(w1646) -> ()
            n476 = call "FGV_GEA2_Ref.vi"("GEA2 Reference In"=w1643, "Action"=enum16{"Set Ref", "Get Ref"}."Set Ref", "Error In"=w1644) -> ("Error Out"=w1640:errorcluster)  [unwired: 11 in, 1 out]
            n477 = call "Time Delay"("error in (no error)"=w1640, "Delay Time (s)"=3.0) -> ("error out"=w1639:errorcluster)  [unwired: 9 in]
            n478 = call "GEA2 Stop.vi"("GEA2 Reference In"=w1637, "Error In"=w1639) -> ("Error Out"=w1638:errorcluster)  [unwired: 13 in]
          }
          event "Stop": Value Change {
            n479 = event-data() -> ()  [unwired: 1 in, 6 out]
          }
        }
        n480 = call "Error_Control_Brass.vi"("Error In"=w1612) -> ("Error Out"=w1614:errorcluster)  [unwired: 14 in]
      }
      n481 = while "Continuous Send Loop" {
        shift-right: [w140] -> _
        shift-left: Cont_Send_States."Run" ("State") -> [w139]
        tunnel: w37 -> [w141]
        tunnel: [w134] -> _
        shift-right: [w132] -> w41
        shift-left: w32 -> [w143]
        stop <- w142 stop-if-true
        # "Continuous Send Loop"
        n482 = Dequeue Element(queue=w141, timeout in ms (-1)=0, error in (no error)=w143) -> (queue out=w135:refnum<queue>, element=w128:T18, timed out?=w136:bool, error out=w131:errorcluster)
        n483 = Select(t=w139, s=w136, f=w128) -> (s? t:f=w138:T18)
        n484 = property on="GEA2 Send" class="Clust (strict)"() -> ("Value"=w130:T3)  [unwired: 2 in, 2 out]
        n485 = case shown="\"Run\", Default" w138 {
          selector: w138 -> [w147 w162]
          tunnel: w131 -> [w149 w164]
          tunnel: [w148 w164] -> w133
          tunnel: [_ TRUE] -> w142
          tunnel: [w147 w162] -> w140
          tunnel: w135 -> [w146 w161]
          tunnel: [w146 w161] -> w134
          tunnel: w130 -> [w145 _]
          frame "Run", Default {
            n486 = case shown="True" "Start Send" {
              tunnel: w149 -> [w150 w153]
              tunnel: [w150 w157] -> w148
              tunnel: w145 -> [_ w155]
              frame False {
              }
              frame True {
                n487 = call "FGV_GEA2_Ref.vi"("Action"=enum16{"Set Ref", "Get Ref"}."Get Ref", "Error In"=w153) -> ("GEA2 Reference Out"=w151:refnum<k24>, "Error Out"=w152:errorcluster)  [unwired: 12 in]
                n488 = call "GEA2MessageFormatter.vi"("Prefix(Send/Recv)"="SEND", "GEA2 Data In"=w155, "Error In"=w152) -> ("Output String"=w156:string, "Error Out"=w160:errorcluster)  [unwired: 11 in]
                n489 = call "GExplorer_Queue_GEA2.vi"("Output String"=w156, "error in (no error)"=w160) -> ("error out"=w158:errorcluster)  [unwired: 13 in]
                n490 = call "GEA2 Send Message.vi"("GEA2 Reference In"=w151, "Input Data"=w155, "Error In"=w158) -> ("Error Out"=w157:errorcluster)  [unwired: 11 in, 1 out]
              }
            }
          }
          frame "Shutdown" {
          }
        }
        n491 = call "Error_Control_Brass.vi"("Error In"=w133) -> ("Error Out"=w132:errorcluster)  [unwired: 14 in]
        n492 = Wait (ms)(milliseconds to wait="Msg Rate (ms)") -> ()  [unwired: 1 out]
      }
      n493 = while "GEA2 Display Loop" {
        tunnel: w67 -> [w385]
        shift-right: [w382] -> _
        shift-left: _ -> [w388]
        shift-right: [w384] -> w96
        shift-left: w31 -> [w392]
        tunnel: w29 -> [w378]
        tunnel: [w376] -> w27
        stop <- w386 stop-if-true
        # "GEA2 Display Loop"
        n494 = Dequeue Element(queue=w385, error in (no error)=w392) -> (element=w391:T20, error out=w387:errorcluster)  [unwired: 1 in, 2 out]
        n495 = Unbundle By Name(w391) -> ("Data"=w389:variant, "State"=w390:enum16{"Add to Log", "Clear", "Shutdown"})
        n496 = case shown="\"Add to Log\", Default" w390 {
          tunnel: w389 -> [w403 _ _]
          tunnel: w388 -> [w406 w411 _]
          tunnel: [w405 w411 ""] -> w383
          tunnel: w387 -> [w404 w412 w416]
          tunnel: [w401 w412 w416] -> w379
          tunnel: [FALSE TRUE FALSE] -> w386
          tunnel: [w393 _ _] -> w377
          frame "Add to Log", Default {
            n497 = Variant To Data(error in=w404, type="", Variant=w403) -> (data=w395:string, error out=w401:errorcluster)
            n498 = String Subset(string=w395, offset (0)=22, length (rest)=7 ("length (rest)")) -> (substring=w396:string)
            n499 = Equal?(x="SEND E5", y=w396) -> (x = y?=w394:bool)
            n500 = case shown="True" w394 {
              tunnel: w406 -> [w409 w410]
              tunnel: [w408 w410] -> w405
              tunnel: w395 -> [w407 _]
              tunnel: [w407 _] -> w393
              frame False {
                n501 = Concatenate Strings(w407, w409) -> (w408:string)
              }
              frame True {
              }
            }
          }
          frame "Shutdown" {
          }
          frame "Clear" {
          }
        }
        "GEA2 Log" <- w383
        n502 = call "Write _To_TXT_File.vi"("refnum"=w378, "text"=w377, "error in"=w379) -> ("refnum out"=w376:refnum<file>, "error out"=w380:errorcluster)  [unwired: 10 in, 1 out]
        n503 = call "Error_Control_Brass.vi"("Error In"=w380) -> ("Error Out"=w384:errorcluster)  [unwired: 14 in]
        n504 = String Subset(string=w383, length (rest)="GEA2 Log Length") -> (substring=w382:string)  [unwired: 1 in]
      }
      n505 = Close File(refnum=w27, error in=w96) -> (error out=w28:errorcluster)  [unwired: 1 out]
      n506 = call "GEA2 Stop.vi"("GEA2 Reference In"=w124, "Error In"=w125) -> ("Error Out"=w108:errorcluster)  [unwired: 13 in]
      n507 = Close File(refnum=w47, error in=w49) -> (error out=w48:errorcluster)  [unwired: 1 out]
      n508 = Merge Errors(w48, w28, w41, w126, w108, w95) -> (w23:errorcluster)
      n509 = Obtain Queue(name (unnamed)="Continuous Send", element data type=Cont_Send_States_Brass."Run" ("State"), error in (no error)=w23) -> (queue out=w46:refnum<queue>, error out=w45:errorcluster)  [unwired: 2 in, 1 out]
      n510 = Obtain Queue(name (unnamed)="ERD Loop", element data type=T22 {"Data"=variant, "State"=enum."Read ERDs"} ("Data"), error in (no error)=w23) -> (queue out=w103:refnum<queue>, error out=w102:errorcluster)  [unwired: 2 in, 1 out]
      n511 = Obtain Queue(name (unnamed)="GEA2", element data type=T20 {"Data"=variant, "State"=enum."Add to Log"} ("Data"), error in (no error)=w23) -> (queue out=w112:refnum<queue>, error out=w111:errorcluster)  [unwired: 2 in, 1 out]
      n512 = Obtain Queue(name (unnamed)="DAQ", element data type=DAQ_States_Brass."Wait for Init" ("States"), error in (no error)=w23) -> (queue out=w98:refnum<queue>, error out=w99:errorcluster)  [unwired: 2 in, 1 out]
      n513 = Release Queue(queue=w46, error in (no error)=w45) -> (error out=w44:errorcluster)  [unwired: 1 in, 2 out]
      n514 = Release Queue(queue=w103, error in (no error)=w102) -> (error out=w91:errorcluster)  [unwired: 1 in, 2 out]
      n515 = Release Queue(queue=w112, error in (no error)=w111) -> (error out=w92:errorcluster)  [unwired: 1 in, 2 out]
      n516 = Release Queue(queue=w98, error in (no error)=w99) -> (error out=w93:errorcluster)  [unwired: 1 in, 2 out]
      n517 = Merge Errors(w44, w91, w92, w93) -> (w90:errorcluster)
      n518 = call "Error_Control_Brass.vi"("Command (Handle Errors)"=Error_Command_Brass."Report Errors", "Error In"=w90) -> ("Error Out"=w83:errorcluster)  [unwired: 13 in]
    }
    frame Error {
    }
  }
  n519 = call <vilib>:"Simple Error Handler.vi"("error in (no error)"=w2) -> ("error out"=→"Error Out":errorcluster)  [unwired: 4 in, 4 out]
